vi "运维调试_五参数.vi"() -> ()   [LabVIEW 2016, in "斯坦道仪器.lvlib"]
uses:
  <vilib>/Utility/miscctls.llb/LVPointTypeDef.ctl
  PLC/PLC.lvlib
panel:
  in  "标样核查":bool
  in  "打开串口":bool
  in  "释放串口":bool
  in  "手动通电":bool
  out "多参数横条运行状态":T1(xcontrol)
  in  "数据区":i32(listbox)
  in  "探头选择":u16(ring)=9 items=["氨氮"=3, "水温"=9, "pH值"=10, "溶解氧"=11, "电导率"=12, "浊度"=13, "叶绿素a"=14, "藻密度"=15, "蓝绿藻"=16, "氧化还原电位"=17, "溶解氧%"=18, "盐度"=19]
  in  "测量数据区读取":bool
  in  "测量数据区":i32(listbox)
  in  "状态告警区读取":bool
  in  "状态告警区":i32(listbox)
  in  "自动校准":bool
  in  "读取KB":bool
  in  "写入KB":bool
  out "B":dbl caption="校准值B:"
  out "K":dbl caption="校准值K:"
  in  "校准区探头选择":u16(ring)=9 items=["氨氮"=3, "水温"=9, "pH值"=10, "溶解氧"=11, "电导率"=12, "浊度"=13, "叶绿素a"=14, "藻密度"=15, "蓝绿藻"=16, "氧化还原电位"=17, "溶解氧%"=18, "盐度"=19]
  in  "停止测量(单探)":bool
  in  "启动测量(单探)":bool
  in  "控制命令区探头选择":u16(ring)=9 items=["氨氮"=3, "水温"=9, "pH值"=10, "溶解氧"=11, "电导率"=12, "浊度"=13, "叶绿素a"=14, "藻密度"=15, "蓝绿藻"=16, "氧化还原电位"=17, "溶解氧%"=18, "盐度"=19]
  in  "同步时间":bool
  in  "初始化(清洗)":bool
  in  "停止测量(全部)":bool
  in  "启动测量(全部)":bool
  in  "关键参数区读取":bool
  in  "关键参数区":i32(listbox)
  in  "传感器参数读取":bool
  in  "传感器区":i32(listbox)
  in  "返回":bool
  in  "设置":bool
  out "运行状态":string
  out "开机状态":bool
  in  "停止":bool
  in  "水样测试":bool
  out "集成报警信息":string
  # "控制命令区"
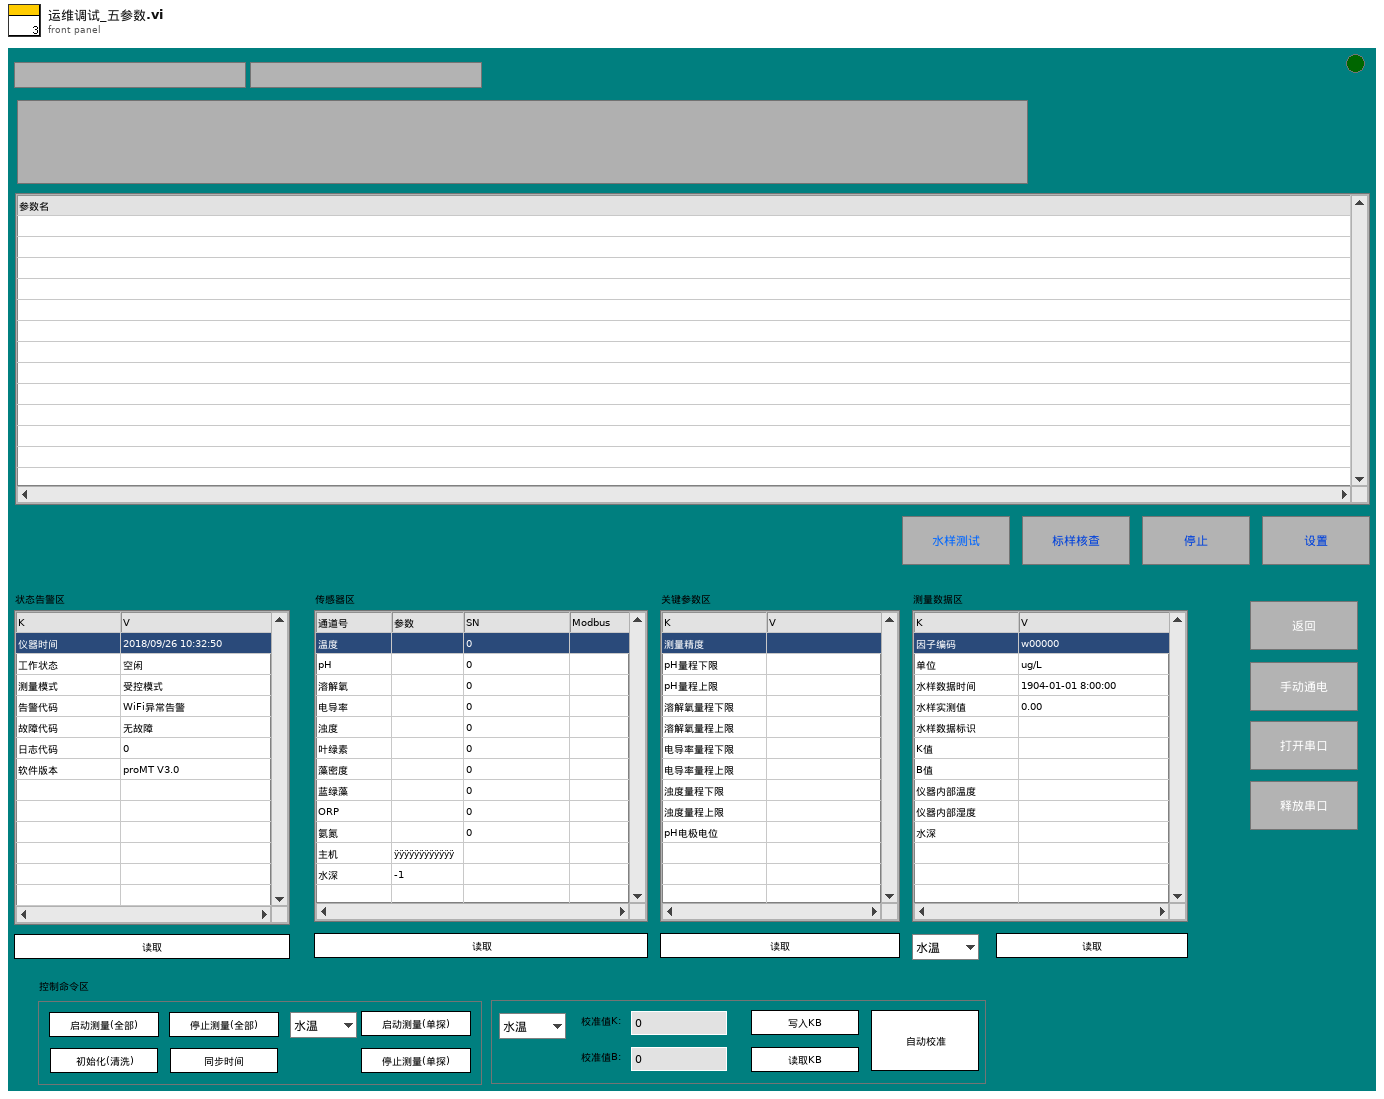
[diagram p1: front panel]
types:
  T1 = cluster{"系统时间":timestamp, "工作状态":u16, "测量模式":u16, "告警代码":enum16{"无告警", "缺试剂告警", "缺水样告警", "缺蒸馏水告警", "缺标液告警", "仪表漏液告警", "标定异常告警", "超量程告警", "加热异常", "低试剂预警", "超上限告警", "超下限告警", "仪表内部其他异常", "滴定异常告警", "电极异常告警", "量程切换告警", "参数设置告警", "PH电极电位异常", "电导率电极异常", "浊度光度异常", "溶解氧电极异常", "溶解氧光强异常", "温度异常告警", "PH异常告警", "溶解氧异常告警", "电导率异常告警", "浊度异常告警", "叶绿素异常告警", "藻密度异常告警", "蓝绿藻异常告警", "ORP异常告警", "氨氮异常告警", "清洁刷异常告警", "SD卡异常告警", "蓝牙异常告警", "Wifi异常告警", "流程异常告警"}, "故障代码":enum16{"无故障", "电机故障", "温度故障", "通讯故障", "滴定故障"}, "日志代码":u16, "软件版本":string}
  T2 = typedef "LVPointTypeDef.ctl" = cluster{"Horizontal":i16, "Vertical":i16}
  T3 = cluster{"时间标识":timestamp, "设备":string, "日志信息":string}
  T4 = enum16{"无告警", "缺试剂告警", "缺水样告警", "缺蒸馏水告警", "缺标液告警", "仪表漏液告警", "标定异常告警", "超量程告警", "加热异常", "低试剂预警", "超上限告警", "超下限告警", "仪表内部其他异常", "滴定异常告警", "电极异常告警", "量程切换告警", "参数设置告警", "PH电极电位异常", "电导率电极异常", "浊度光度异常", "溶解氧电极异常", "溶解氧光强异常", "温度异常告警", "PH异常告警", "溶解氧异常告警", "电导率异常告警", "浊度异常告警", "叶绿素异常告警", "藻密度异常告警", "蓝绿藻异常告警", "ORP异常告警", "氨氮异常告警", "清洁刷异常告警", "SD卡异常告警", "蓝牙异常告警", "Wifi异常告警", "流程异常告警"}
  T5 = cluster{"水温":dbl, "pH":dbl, "DO":dbl, "Cond":dbl, "Turb":dbl, "叶绿素":dbl, "藻密度":dbl, "蓝绿藻":dbl, "ORP":dbl, "NH3N":dbl}
  T6 = cluster{"因子编码":string, "单位":string, "标样参考值":sgl, "水样数据时间":timestamp, "水样实测值":sgl, "水样数据标识":string, "K":sgl, "B":sgl, "T":sgl, "H":sgl, "水深":sgl}
  T7 = enum8{"Enabled", "Disabled", "Disabled and Grayed Out"}
  T8 = cluster{"测量模式":enum16{"待机", "水样测试", "标样核查", "零点核查", "跨度核查", "空白测试", "平行样测试", "加标回收", "空白校准", "标样校准", "初始化（清洗）"}, "数据标记表":string, "测量时间":dbl}
  T9 = cluster{"测量模式":enum16{"待机", "水样测试", "标样核查", "零点核查", "跨度核查", "空白测试", "平行样测试", "加标回收", "空白校准", "标样校准", "初始化（清洗）"}, "数据标记表":string, "输出参数":cluster{"水温":bool, "pH":bool, "DO":bool, "浊度":bool, "电导率":bool, "保存组数":dbl}}
  T10 = enum16{"待机", "水样测试", "标样核查", "零点核查", "跨度核查", "空白测试", "平行样测试", "加标回收", "空白校准", "标样校准", "初始化（清洗）"}
  T11 = cluster{"starting address":u16, "holding register value":u16}
  T12 = enum16{"idle", "init", "读状态", "读参数", "多个写入", "单个写入", "线圈写入"}
  T13 = enum32{"Bad", "Idle", "Run top level", "Running"}
  T14 = cluster{"水温":bool, "pH":bool, "DO":bool, "浊度":bool, "电导率":bool, "保存组数":dbl}
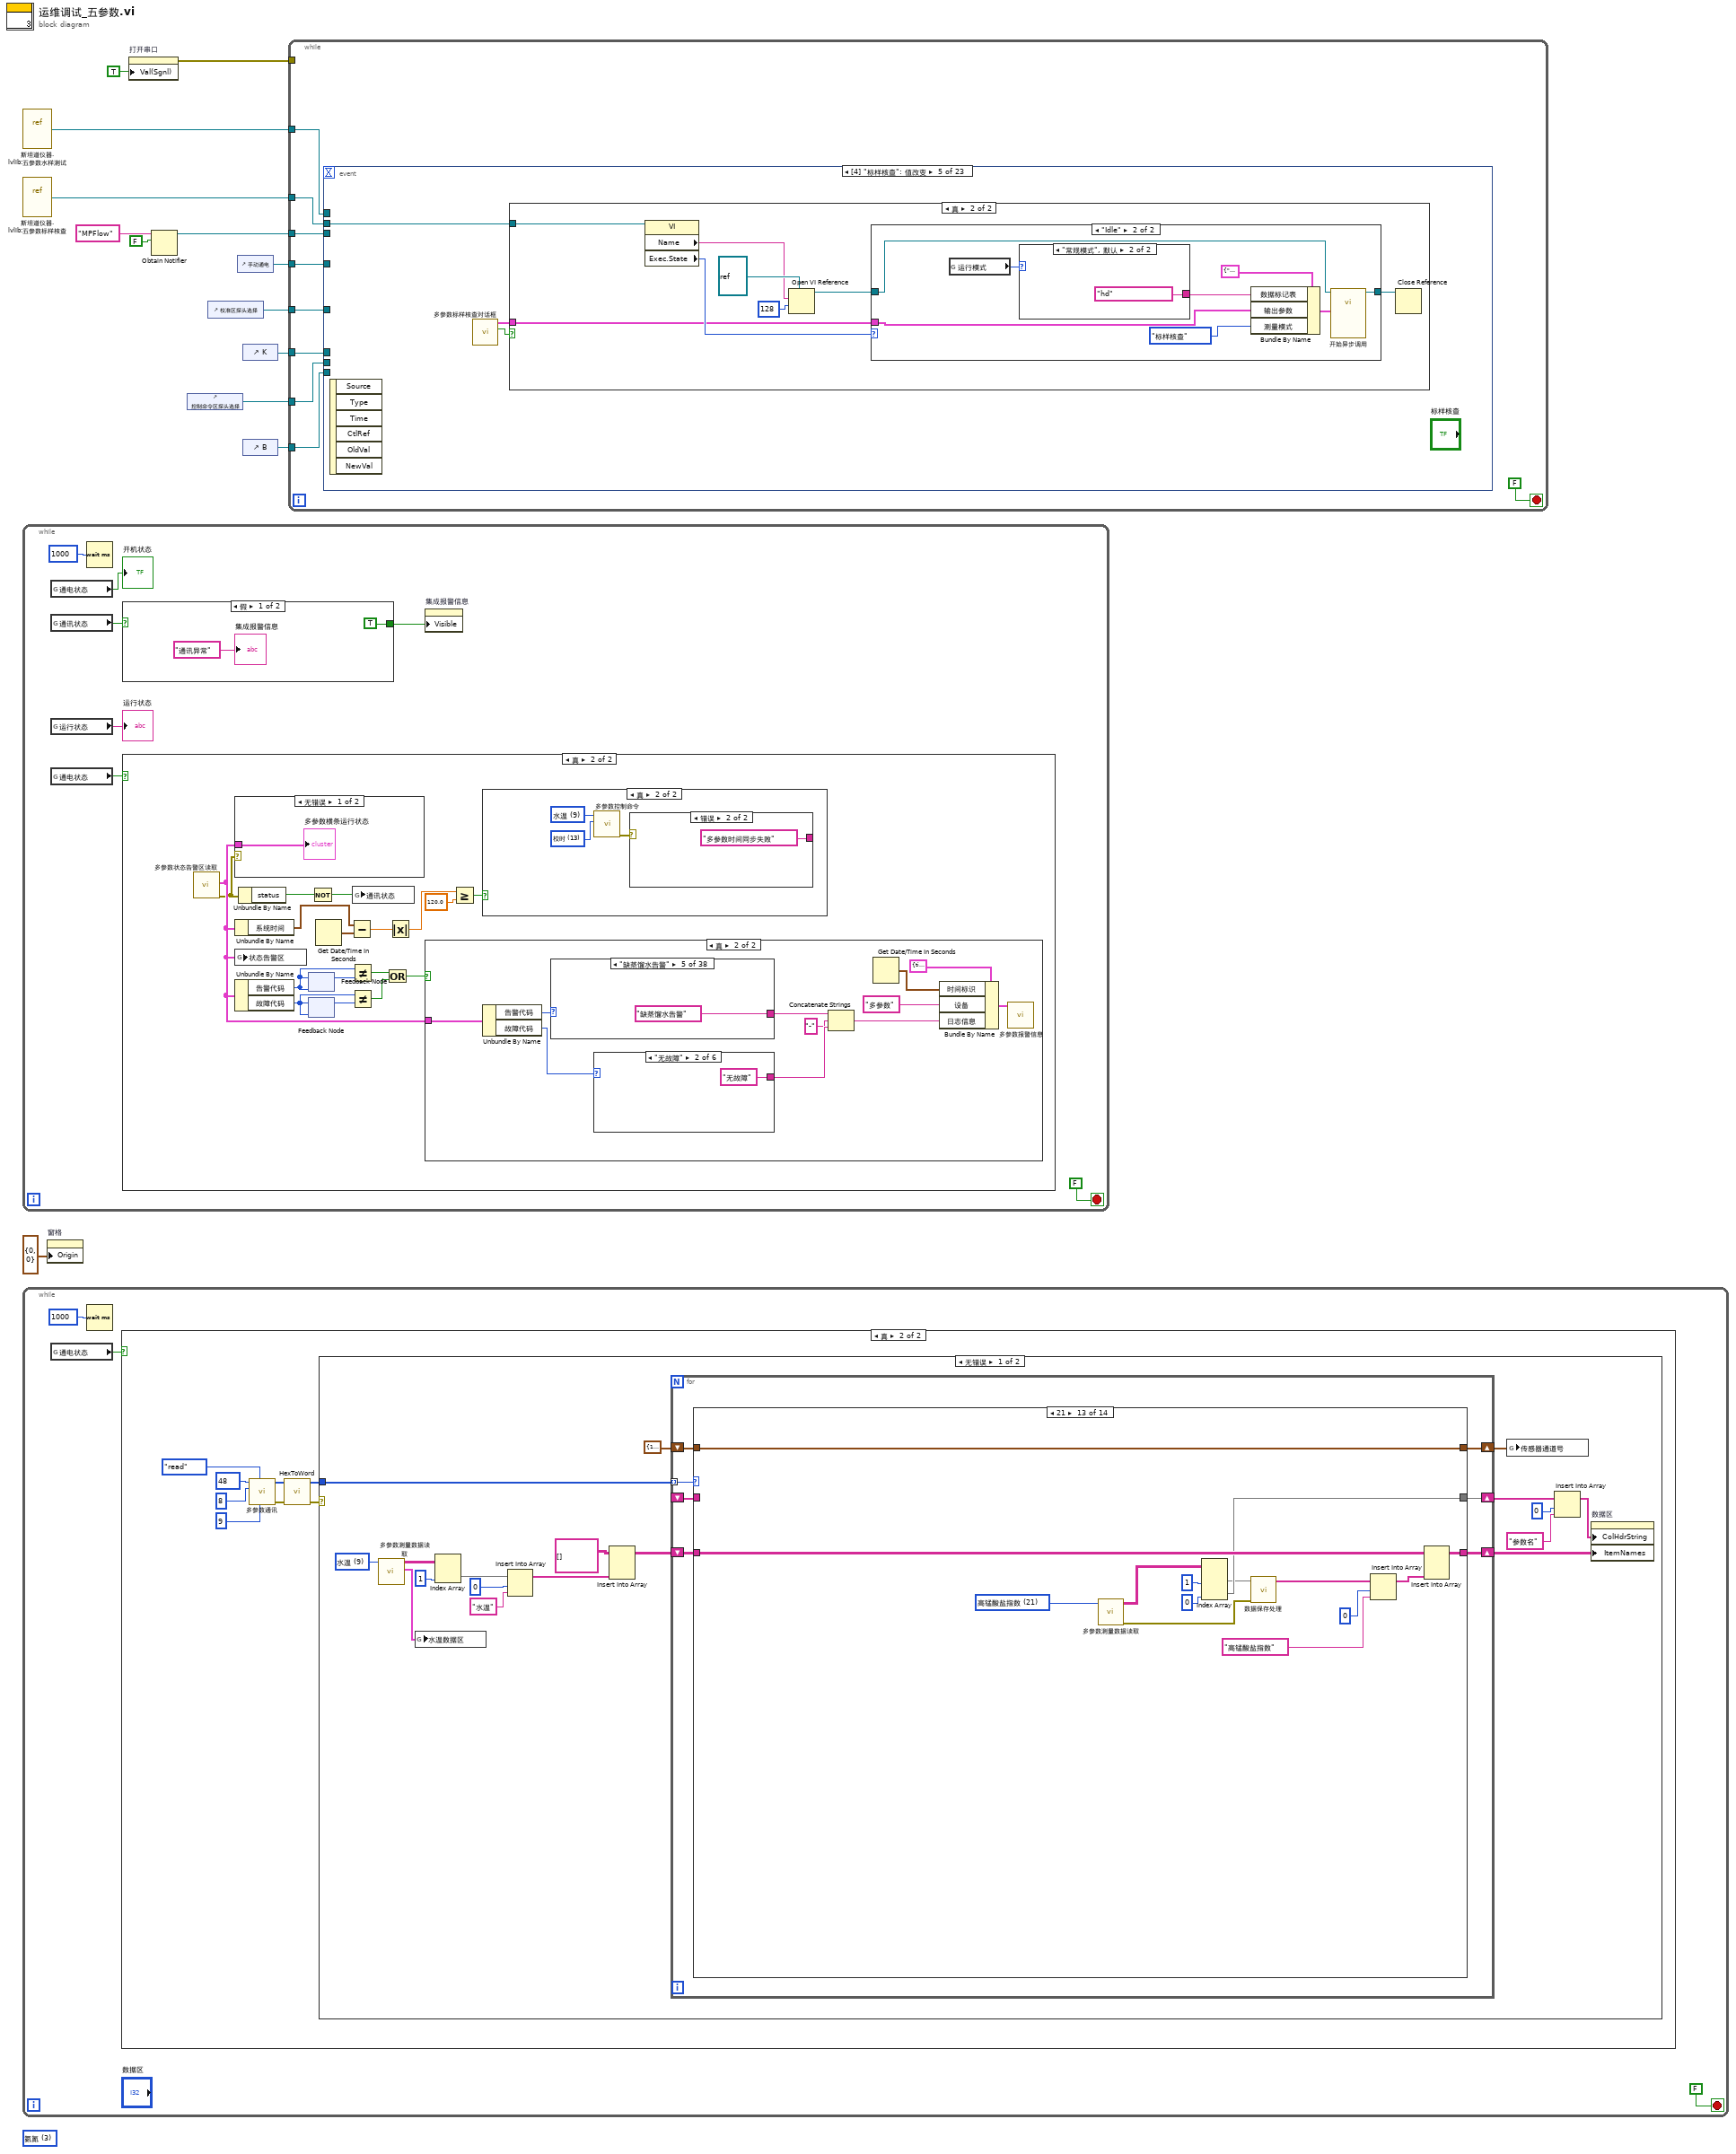
[diagram p0: block diagram]
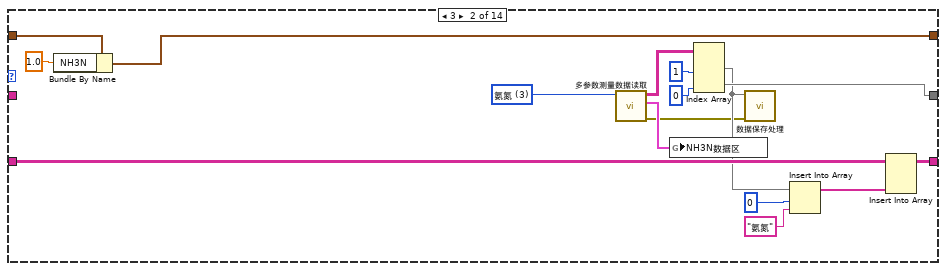
[diagram p4: hidden frame]
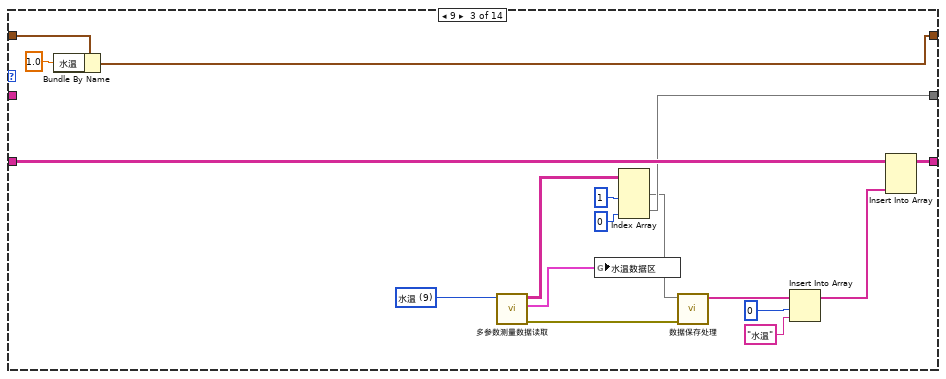
[diagram p5: hidden frame]
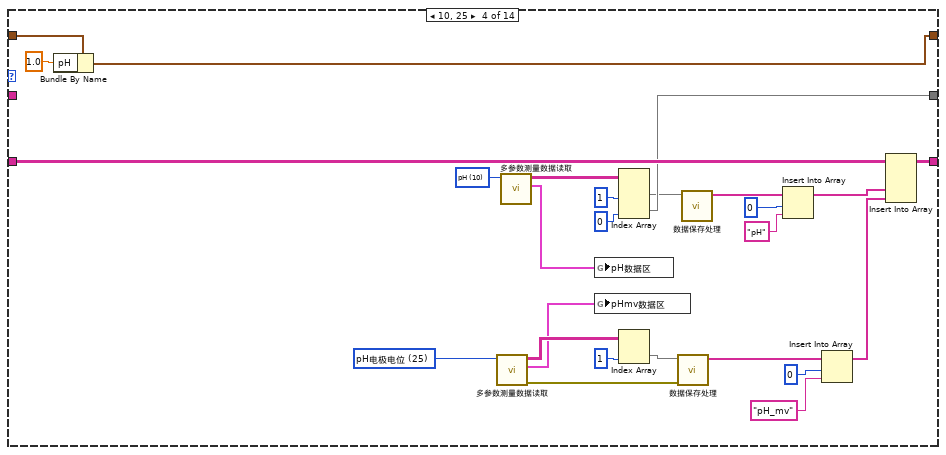
[diagram p6: hidden frame]
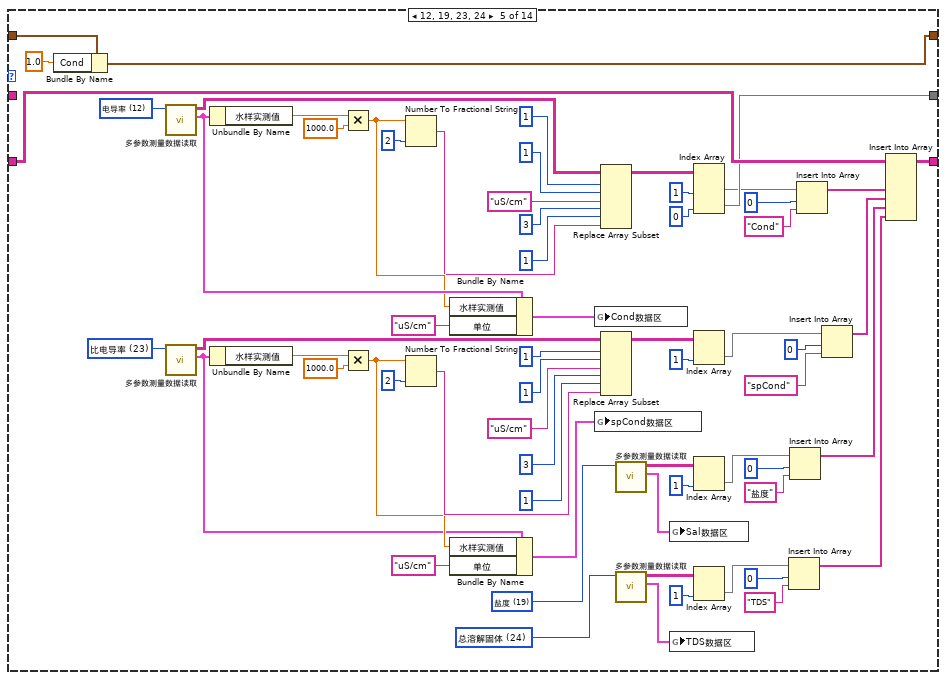
[diagram p7: hidden frame]
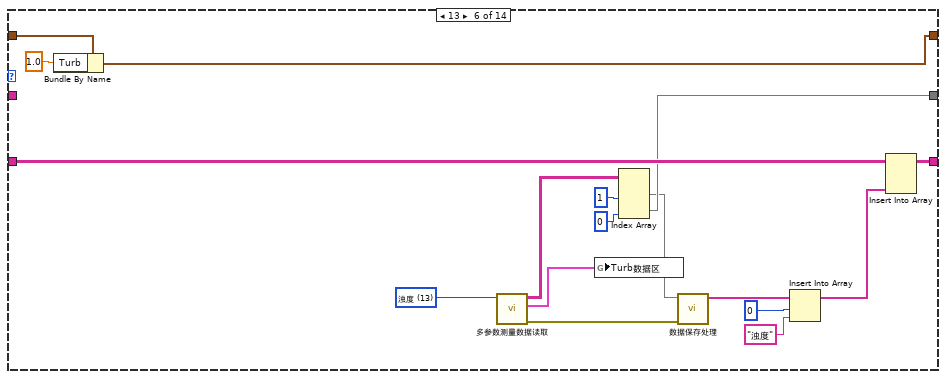
[diagram p8: hidden frame]
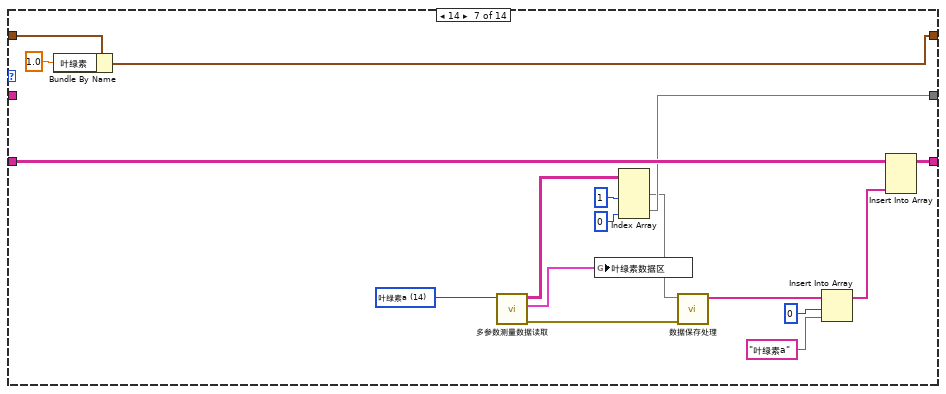
[diagram p9: hidden frame]
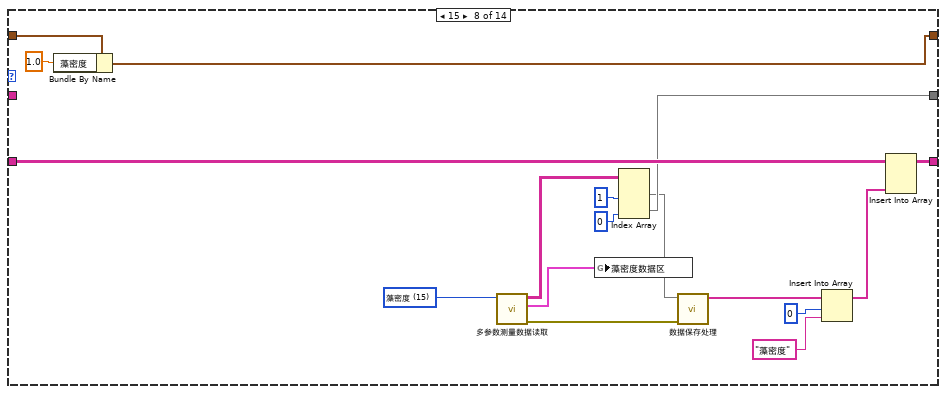
[diagram p10: hidden frame]
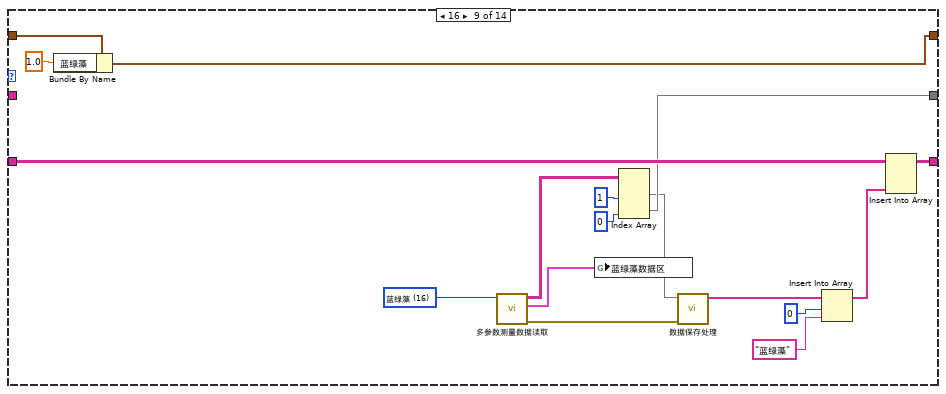
[diagram p11: hidden frame]
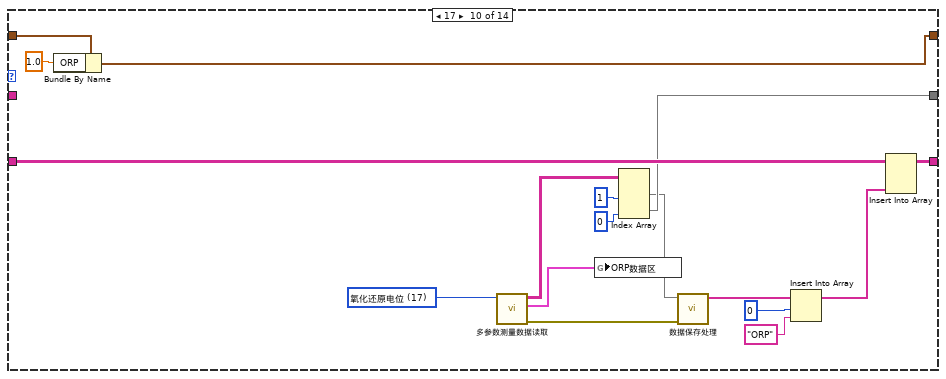
[diagram p12: hidden frame]
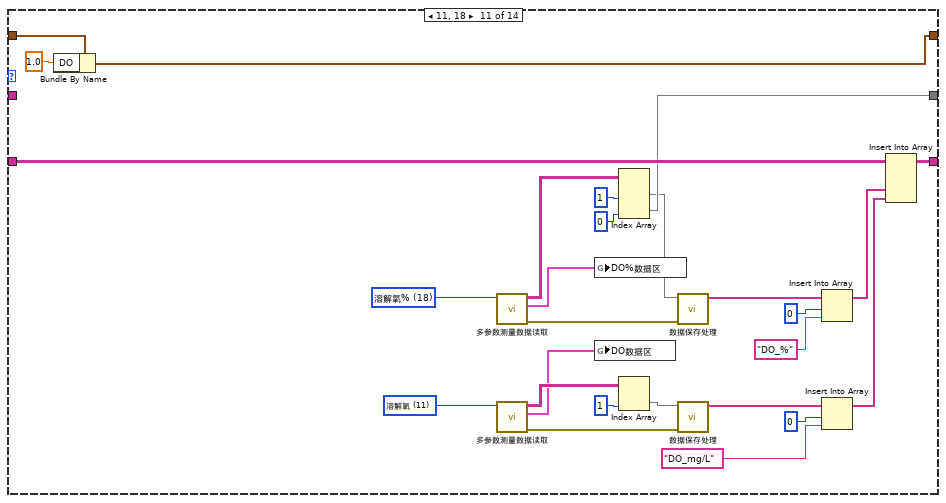
[diagram p13: hidden frame]
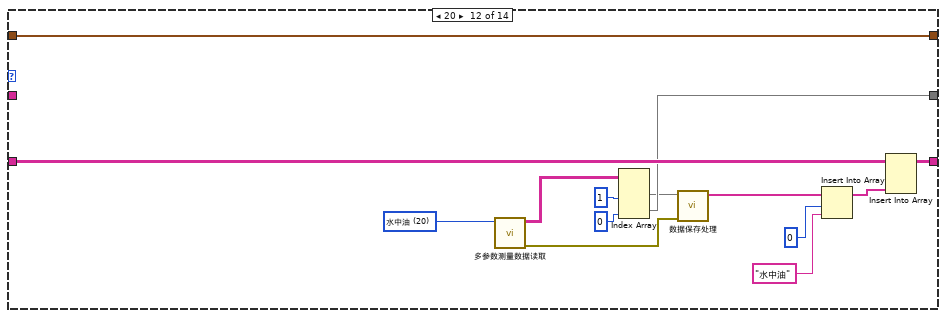
[diagram p14: hidden frame]
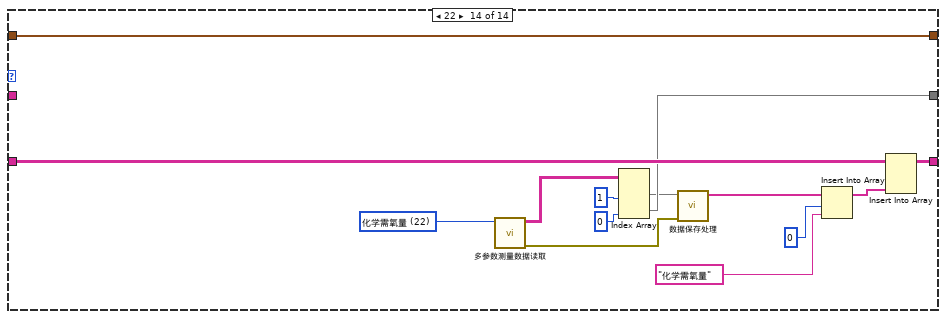
[diagram p15: hidden frame]
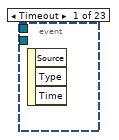
[diagram p17: hidden frame]
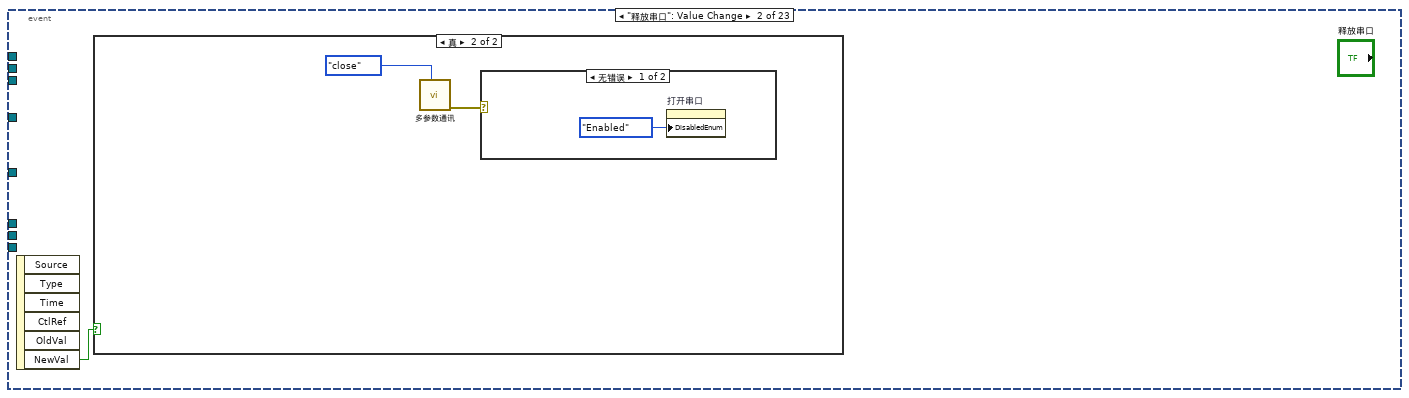
[diagram p18: hidden frame]
diagram:
  (unwired) u16 3 items=["氨氮"=3, "水温"=9, "pH"=10, "溶解氧"=11, "电导率"=12, "浊度"=13, "叶绿素a"=14, "藻密度"=15, "蓝绿藻"=16, "氧化还原电位"=17, "溶解氧%"=18, "盐度"=19, "水中油"=20, "高锰酸盐指数"=21, "化学需氧量"=22, "比电导率"=23, "总溶解固体"=24, "pH电极电位"=25] ("下拉列表")
  n1 = vi-ref "斯坦道仪器.lvlib:五参数水样测试.vi"() -> (w10:refnum<vi>)
  n2 = vi-ref "斯坦道仪器.lvlib:五参数标样核查.vi"() -> (w1:refnum<vi>)
  n3 = while {
    stop <- FALSE stop-if-true
    n4 = global read "多参数全局变量.vi" "通电状态"() -> (→"开机状态":bool)
    n5 = global read "多参数全局变量.vi" "通讯状态"() -> (w18:bool)
    n6 = global read "多参数全局变量.vi" "运行状态"() -> (→"运行状态":string)
    n7 = global read "多参数全局变量.vi" "通电状态"() -> (w14:bool)
    n8 = Wait (ms)(milliseconds to wait=u32 1000 ("等待时间（毫秒）")) -> ()  [unwired: 1 out]
    n9 = case shown="假" w18 {
      tunnel: [TRUE ("可见") _] -> w17
      frame False {
        "集成报警信息" <- "通讯异常" ("集成报警信息")
      }
      frame True {
      }
    }
    n10 = case shown="真" w14 {
      frame False {
      }
      frame True {
        n11 = call "多参数状态告警区读取.vi"() -> ("error out"=w21:errorcluster, "状态告警块"=w28:T1)  [unwired: 9 in, 1 out]
        n12 = case shown="无错误" w21 {
          tunnel: w28 -> [w38 _]
          frame No Error {
            "多参数横条运行状态" <- w38
          }
          frame Error {
          }
        }
        n13 = Unbundle By Name(w28) -> ("系统时间"=w27:timestamp)
        n14 = global write "多参数全局变量.vi" "状态告警区"(w28) -> ()
        n15 = Unbundle By Name(w28) -> ("告警代码"=w36:T4, "故障代码"=w34:enum16{"无故障", "电机故障", "温度故障", "通讯故障", "滴定故障"})
        n16 = Unbundle By Name(w21) -> ("status"=w30:bool)
        n17 = feedback #1(w36) -> (w37:T4)
        n18 = feedback-in #1(w36) -> ()
        n19 = feedback #2(w34) -> (w35:enum16{"无故障", "电机故障", "温度故障", "通讯故障", "滴定故障"})
        n20 = feedback-in #2(w34) -> ()
        n21 = Not(x=w30) -> (.not. x?=w29:bool)
        n22 = Get Date/Time In Seconds() -> (seconds since 1Jan1904=w26:timestamp)
        n23 = Subtract(x=w27, y=w26) -> (x-y=w25:dbl)
        n24 = Not Equal?(x=w36, y=w37) -> (x != y?=w32:bool)
        n25 = Not Equal?(x=w34, y=w35) -> (x != y?=w33:bool)
        n26 = global write "多参数全局变量.vi" "通讯状态"(w29) -> ()
        n27 = Or(x=w32, y=w33) -> (x .or. y?=w31:bool)
        n28 = Absolute Value(x=w25) -> (abs(x)=w24:dbl)
        n29 = case shown="真" w31 {
          tunnel: w28 -> [_ w54]
          frame False {
          }
          frame True {
            n30 = Unbundle By Name(w54) -> ("告警代码"=w53:T4, "故障代码"=w52:enum16{"无故障", "电机故障", "温度故障", "通讯故障", "滴定故障"})
            n31 = case shown="\"缺蒸馏水告警\"" w53 {
              selector: w53 -> [w65 _ _ _ _ _ _ _ _ _ _ _ _ _ _ _ _ _ _ _ _ _ _ _ _ _ _ _ _ _ _ _ _ _ _ _ _ _]
              tunnel: [w64 "无告警" "缺试剂告警" "缺水样告警" "缺蒸馏水告警" "缺标液告警" "仪表漏液告警" "标定异常告警" "超量程告警" "加热异常" "低试剂预警" "超上限告警" "超下限告警" "仪表内部其他异常" "滴定异常告警" "电极异常告警" "量程切换告警" "参数设置告警" "PH电极电位异常" "电导率电极异常" "浊度光度异常" "溶解氧电极异常" "溶解氧光强异常" "温度异常告警" "PH异常告警" "溶解氧异常告警" "电导率异常告警" "浊度异常告警" "叶绿素异常告警" "藻密度异常告警" "蓝绿藻异常告警" "ORP异常告警" "氨氮异常告警" "清洁刷异常告警" "SD卡异常告警" "蓝牙异常告警" "WiFi异常告警" "流程异常告警"] -> w51
              frame Default {
                n32 = Format Into String(format string="%d" ("格式字符串"), initial string="未知" ("工作状态"), w65) -> (resulting string=w64:string)  [unwired: 1 in, 1 out]
              }
              frame "无告警" {
              }
              frame "缺试剂告警" {
              }
              frame "缺水样告警" {
              }
              frame "缺蒸馏水告警" {
              }
              frame "缺标液告警" {
              }
              frame "仪表漏液告警" {
              }
              frame "标定异常告警" {
              }
              frame "超量程告警" {
              }
              frame "加热异常" {
              }
              frame "低试剂预警" {
              }
              frame "超上限告警" {
              }
              frame "超下限告警" {
              }
              frame "仪表内部其他异常" {
              }
              frame "滴定异常告警" {
              }
              frame "电极异常告警" {
              }
              frame "量程切换告警" {
              }
              frame "参数设置告警" {
              }
              frame "PH电极电位异常" {
              }
              frame "电导率电极异常" {
              }
              frame "浊度光度异常" {
              }
              frame "溶解氧电极异常" {
              }
              frame "溶解氧光强异常" {
              }
              frame "温度异常告警" {
              }
              frame "PH异常告警" {
              }
              frame "溶解氧异常告警" {
              }
              frame "电导率异常告警" {
              }
              frame "浊度异常告警" {
              }
              frame "叶绿素异常告警" {
              }
              frame "藻密度异常告警" {
              }
              frame "蓝绿藻异常告警" {
              }
              frame "ORP异常告警" {
              }
              frame "氨氮异常告警" {
              }
              frame "清洁刷异常告警" {
              }
              frame "SD卡异常告警" {
              }
              frame "蓝牙异常告警" {
              }
              frame "Wifi异常告警" {
              }
              frame "流程异常告警" {
              }
            }
            n33 = case shown="\"无故障\"" w52 {
              selector: w52 -> [w56 _ _ _ _ _]
              tunnel: [w55 "无故障" "电机故障" "温度故障" "通讯故障" "滴定故障"] -> w50
              frame Default {
                n34 = Format Into String(format string="%d" ("格式字符串"), initial string="未知" ("工作状态"), w56) -> (resulting string=w55:string)  [unwired: 1 in, 1 out]
              }
              frame "无故障" {
              }
              frame "电机故障" {
              }
              frame "温度故障" {
              }
              frame "通讯故障" {
              }
              frame "滴定故障" {
              }
            }
            n35 = Concatenate Strings(w51, "-" ("字符串"), w50) -> (w46:string)
            n36 = Get Date/Time In Seconds() -> (seconds since 1Jan1904=w45:timestamp)
            n37 = Bundle By Name(cluster=T3 {"时间标识"=timestamp(0 s since 1904-01-01), "设备"="", "日志信息"=""} ("data in"), "时间标识"=w45, "设备"="多参数", "日志信息"=w46) -> (w47:T3)
            n38 = call "多参数报警信息.vi"("data in"=w47) -> ()  [unwired: 10 in, 1 out]
          }
        }
        n39 = Greater Or Equal?(x=w24, y=120.0) -> (x >= y?=w23:bool)
        n40 = case shown="真" w23 {
          frame False {
          }
          frame True {
            w39 = u16 13 items=["启动测量（全部）"=1, "初始化（清洗）"=10, "停止测量（全部）"=11, "校时"=13, "启动测量（单个传感器）"=19, "停止测量（单个传感器）"=20] ("控制命令")
            w40 = u16 9 items=["氨氮"=3, "水温"=9, "pH值"=10, "溶解氧"=11, "电导率"=12, "浊度"=13, "叶绿素a"=14, "藻密度"=15, "蓝绿藻"=16, "氧化还原电位"=17, "溶解氧%"=18, "盐度"=19] ("站号")
            n41 = call "多参数控制命令.vi"("控制命令"=w39, "站号"=w40) -> ("error out"=w41:errorcluster)  [unwired: 9 in]
            n42 = case shown="错误" w41 {
              tunnel: ["多参数时间同步成功" ("消息") "多参数时间同步失败" ("消息")] -> _
              frame No Error {
              }
              frame Error {
              }
            }
          }
        }
      }
    }
    n43 = property on="集成报警信息" class="Str"("Visible"=w17) -> ()  [unwired: 2 in, 2 out]
  }
  n44 = while {
    stop <- FALSE stop-if-true
    n45 = global read "多参数全局变量.vi" "通电状态"() -> (w107:bool)
    n46 = Wait (ms)(milliseconds to wait=u32 1000 ("等待时间（毫秒）")) -> ()  [unwired: 1 out]
    n47 = case shown="真" w107 {
      frame False {
      }
      frame True {
        n48 = call "多参数通讯.vi"("Slave ID"=u8 9, "STEP"=enum16{"open", "read", "write", "close"}."read", "quantity"=u16 8, "starting address"=u16 48) -> ("error out"=w112:errorcluster, "Registers"=w113:u16[])  [unwired: 5 in, 1 out]
        n49 = call "HexToWord.vi"("数组"=w113) -> ("WORD"=w116:u16[])  [unwired: 10 in]
        n50 = case shown="无错误" w112 {
          tunnel: w116 -> [w131 _]
          frame No Error {
            w128 = u16 9 items=["氨氮"=3, "水温"=9, "pH"=10, "溶解氧"=11, "电导率"=12, "浊度"=13, "叶绿素a"=14, "藻密度"=15, "蓝绿藻"=16, "氧化还原电位"=17, "溶解氧%"=18, "盐度"=19, "水中油"=20, "高锰酸盐指数"=21, "化学需氧量"=22, "比电导率"=23, "总溶解固体"=24, "pH电极电位"=25] ("下拉列表")
            n51 = call "多参数测量数据读取.vi"("探头选择"=w128) -> ("测量数据块"=w117:T6, "添加的数组"=w127:string[][])  [unwired: 8 in, 1 out]
            n52 = global write "多参数全局变量.vi" "水温数据区"(w117) -> ()
            n53 = Index Array(array=w127, index (col)=1 ("禁用的索引 (列)")) -> (element=w122:string[])  [unwired: 1 in]
            n54 = Insert Into Array(array=w122, index=0 ("索引"), new element="水温") -> (w124:string[])
            n55 = Insert Into Array(array=string[][] [] ("子数组"), new element=w124) -> (w120:string[][])  [unwired: 2 in]
            n56 = for {
              tunnel: w131 -> [w141] mode=indexing
              shift-right: [w139] -> w129
              shift-left: w120 -> [w140]
              shift-right: [w138] -> w130
              shift-left: _ -> [w137]
              shift-right: [w136] -> w118
              shift-left: T5 {"水温"=1.0, "pH"=0.0, "DO"=0.0, "Cond"=0.0, "Turb"=0.0, "叶绿素"=0.0, "藻密度"=0.0, "蓝绿藻"=0.0, "ORP"=0.0, "NH3N"=0.0} ("传感器通道号") -> [w135]
              n57 = case shown="21" w141 {
                tunnel: w140 -> [w144 w156 w173 w199 w265 w281 w298 w315 w332 w349 w376 w390 w404 w418]
                tunnel: [w144 w155 w172 w198 w264 w280 w297 w314 w331 w348 w375 w389 w403 w417] -> w139
                tunnel: [w143 w153 w170 w196 w262 w278 w295 w312 w329 w346 w373 w387 w401 w415] -> w138
                tunnel: w137 -> [w143 _ _ _ _ _ _ _ _ _ _ _ _ _]
                tunnel: [w142 w148 w165 w185 w238 w273 w290 w307 w324 w341 w362 w384 w398 w412] -> w136
                tunnel: w135 -> [w142 w150 w167 w187 w239 w274 w291 w308 w325 w342 w363 w384 w398 w412]
                frame 0, Default {
                }
                frame 3 {
                  w160 = u16 3 items=["氨氮"=3, "水温"=9, "pH"=10, "溶解氧"=11, "电导率"=12, "浊度"=13, "叶绿素a"=14, "藻密度"=15, "蓝绿藻"=16, "氧化还原电位"=17, "溶解氧%"=18, "盐度"=19, "水中油"=20, "高锰酸盐指数"=21, "化学需氧量"=22, "比电导率"=23, "总溶解固体"=24, "pH电极电位"=25] ("下拉列表")
                  n58 = Bundle By Name(cluster=w150, "NH3N"=1.0) -> (w148:T5)
                  n59 = call "多参数测量数据读取.vi"("探头选择"=w160) -> ("error out"=w145:errorcluster, "测量数据块"=w147:T6, "添加的数组"=w159:string[][])  [unwired: 8 in]
                  n60 = global write "多参数全局变量.vi" "NH3N数据区"(w147) -> ()
                  n61 = Index Array(array=w159, index (col) #1=1 ("禁用的索引 (列)"), index (col) #2=0 ("禁用的索引 (列)")) -> (element #1=w146:string[], element #2=w153:string[])  [unwired: 2 in]
                  n62 = call "数据保存处理.vi"("error in (no error)"=w145, "数组"=w146) -> ()  [unwired: 8 in, 2 out]
                  n63 = Insert Into Array(array=w146, index=0 ("索引"), new element="氨氮") -> (w154:string[])
                  n64 = Insert Into Array(array=w156, new element=w154) -> (w155:string[][])  [unwired: 2 in]
                }
                frame 9 {
                  w177 = u16 9 items=["氨氮"=3, "水温"=9, "pH"=10, "溶解氧"=11, "电导率"=12, "浊度"=13, "叶绿素a"=14, "藻密度"=15, "蓝绿藻"=16, "氧化还原电位"=17, "溶解氧%"=18, "盐度"=19, "水中油"=20, "高锰酸盐指数"=21, "化学需氧量"=22, "比电导率"=23, "总溶解固体"=24, "pH电极电位"=25] ("下拉列表")
                  n65 = Bundle By Name(cluster=w167, "水温"=1.0) -> (w165:T5)
                  n66 = call "多参数测量数据读取.vi"("探头选择"=w177) -> ("error out"=w161:errorcluster, "测量数据块"=w164:T6, "添加的数组"=w176:string[][])  [unwired: 8 in]
                  n67 = global write "多参数全局变量.vi" "水温数据区"(w164) -> ()
                  n68 = Index Array(array=w176, index (col) #1=1 ("禁用的索引 (列)"), index (col) #2=0 ("禁用的索引 (列)")) -> (element #1=w163:string[], element #2=w170:string[])  [unwired: 2 in]
                  n69 = call "数据保存处理.vi"("error in (no error)"=w161, "数组"=w163) -> ("数组 2"=w162:string[])  [unwired: 8 in, 1 out]
                  n70 = Insert Into Array(array=w162, index=0 ("索引"), new element="水温") -> (w171:string[])
                  n71 = Insert Into Array(array=w173, new element=w171) -> (w172:string[][])  [unwired: 2 in]
                }
                frame 10, 25 {
                  w189 = u16 25 items=["氨氮"=3, "水温"=9, "pH"=10, "溶解氧"=11, "电导率"=12, "浊度"=13, "叶绿素a"=14, "藻密度"=15, "蓝绿藻"=16, "氧化还原电位"=17, "溶解氧%"=18, "盐度"=19, "水中油"=20, "高锰酸盐指数"=21, "化学需氧量"=22, "比电导率"=23, "总溶解固体"=24, "pH电极电位"=25] ("下拉列表")
                  w203 = u16 10 items=["氨氮"=3, "水温"=9, "pH"=10, "溶解氧"=11, "电导率"=12, "浊度"=13, "叶绿素a"=14, "藻密度"=15, "蓝绿藻"=16, "氧化还原电位"=17, "溶解氧%"=18, "盐度"=19, "水中油"=20, "高锰酸盐指数"=21, "化学需氧量"=22, "比电导率"=23, "总溶解固体"=24, "pH电极电位"=25] ("下拉列表")
                  n72 = Bundle By Name(cluster=w187, "pH"=1.0) -> (w185:T5)
                  n73 = call "多参数测量数据读取.vi"("探头选择"=w189) -> ("error out"=w182:errorcluster, "测量数据块"=w183:T6, "添加的数组"=w190:string[][])  [unwired: 8 in]
                  n74 = call "多参数测量数据读取.vi"("探头选择"=w203) -> ("测量数据块"=w184:T6, "添加的数组"=w202:string[][])  [unwired: 8 in, 1 out]
                  n75 = global write "多参数全局变量.vi" "pH数据区"(w184) -> ()
                  n76 = global write "多参数全局变量.vi" "pHmv数据区"(w183) -> ()
                  n77 = Index Array(array=w202, index (col) #1=1 ("禁用的索引 (列)"), index (col) #2=0 ("禁用的索引 (列)")) -> (element #1=w179:string[], element #2=w196:string[])  [unwired: 2 in]
                  n78 = Index Array(array=w190, index (col)=1 ("禁用的索引 (列)")) -> (element=w181:string[])  [unwired: 1 in]
                  n79 = call "数据保存处理.vi"("error in (no error)"=w182, "数组"=w181) -> ("数组 2"=w180:string[])  [unwired: 8 in, 1 out]
                  n80 = call "数据保存处理.vi"("数组"=w179) -> ("数组 2"=w178:string[])  [unwired: 9 in, 1 out]
                  n81 = Insert Into Array(array=w178, index=0 ("索引"), new element="pH") -> (w197:string[])
                  n82 = Insert Into Array(array=w180, index=0 ("索引"), new element="pH_mv") -> (w188:string[])
                  n83 = Insert Into Array(array=w199, new element #1=w197, new element #2=w188) -> (w198:string[][])  [unwired: 2 in]
                }
                frame 12, 19, 23, 24 {
                  w242 = u16 24 items=["氨氮"=3, "水温"=9, "pH"=10, "溶解氧"=11, "电导率"=12, "浊度"=13, "叶绿素a"=14, "藻密度"=15, "蓝绿藻"=16, "氧化还原电位"=17, "溶解氧%"=18, "盐度"=19, "水中油"=20, "高锰酸盐指数"=21, "化学需氧量"=22, "比电导率"=23, "总溶解固体"=24, "pH电极电位"=25] ("下拉列表")
                  w254 = u16 19 items=["氨氮"=3, "水温"=9, "pH"=10, "溶解氧"=11, "电导率"=12, "浊度"=13, "叶绿素a"=14, "藻密度"=15, "蓝绿藻"=16, "氧化还原电位"=17, "溶解氧%"=18, "盐度"=19, "水中油"=20, "高锰酸盐指数"=21, "化学需氧量"=22, "比电导率"=23, "总溶解固体"=24, "pH电极电位"=25] ("下拉列表")
                  w256 = u16 23 items=["氨氮"=3, "水温"=9, "pH"=10, "溶解氧"=11, "电导率"=12, "浊度"=13, "叶绿素a"=14, "藻密度"=15, "蓝绿藻"=16, "氧化还原电位"=17, "溶解氧%"=18, "盐度"=19, "水中油"=20, "高锰酸盐指数"=21, "化学需氧量"=22, "比电导率"=23, "总溶解固体"=24, "pH电极电位"=25] ("下拉列表")
                  w268 = u16 12 items=["氨氮"=3, "水温"=9, "pH"=10, "溶解氧"=11, "电导率"=12, "浊度"=13, "叶绿素a"=14, "藻密度"=15, "蓝绿藻"=16, "氧化还原电位"=17, "溶解氧%"=18, "盐度"=19, "水中油"=20, "高锰酸盐指数"=21, "化学需氧量"=22, "比电导率"=23, "总溶解固体"=24, "pH电极电位"=25] ("下拉列表")
                  n84 = Bundle By Name(cluster=w239, "Cond"=1.0 ("DO")) -> (w238:T5)
                  n85 = call "多参数测量数据读取.vi"("探头选择"=w268) -> ("测量数据块"=w228:T6, "添加的数组"=w235:string[][])  [unwired: 8 in, 1 out]
                  n86 = call "多参数测量数据读取.vi"("探头选择"=w256) -> ("测量数据块"=w206:T6, "添加的数组"=w207:string[][])  [unwired: 8 in, 1 out]
                  n87 = Unbundle By Name(w228) -> ("水样实测值"=w230:sgl)
                  n88 = Unbundle By Name(w206) -> ("水样实测值"=w213:sgl)
                  n89 = Multiply(x=w230, y=sgl 1000.0) -> (x*y=w223:sgl)
                  n90 = Multiply(x=w213, y=sgl 1000.0) -> (x*y=w218:sgl)
                  n91 = Number To Fractional String(number=w223, precision (6)=i16 2 ("精度(6)")) -> (F-format string=w221:string)  [unwired: 2 in]
                  n92 = Number To Fractional String(number=w218, precision (6)=i16 2 ("精度(6)")) -> (F-format string=w220:string)  [unwired: 2 in]
                  n93 = Bundle By Name(cluster=w228, "水样实测值"=w223, "单位"="uS/cm" ("新元素/子数组")) -> (w226:T6)
                  n94 = Bundle By Name(cluster=w206, "水样实测值"=w218, "单位"="uS/cm" ("新元素/子数组")) -> (w205:T6)
                  n95 = global write "多参数全局变量.vi" "Cond数据区"(w226) -> ()
                  n96 = global write "多参数全局变量.vi" "spCond数据区"(w205) -> ()
                  n97 = Replace Array Subset(array=w235, new element #1="uS/cm" ("新元素/子数组"), index (row) #1=1 ("索引 (行)"), index (col) #1=1 ("禁用的索引 (列)"), new element #2=w221, index (row) #2=3 ("索引 (行)"), index (col) #2=1 ("禁用的索引 (列)")) -> (w231:string[][])
                  n98 = Replace Array Subset(array=w207, new element #1="uS/cm" ("新元素/子数组"), index (row) #1=1 ("索引 (行)"), index (col) #1=1 ("禁用的索引 (列)"), new element #2=w220, index (row) #2=3 ("索引 (行)"), index (col) #2=1 ("禁用的索引 (列)")) -> (w212:string[][])
                  n99 = call "多参数测量数据读取.vi"("探头选择"=w254) -> ("测量数据块"=w237:T6, "添加的数组"=w253:string[][])  [unwired: 8 in, 1 out]
                  n100 = call "多参数测量数据读取.vi"("探头选择"=w242) -> ("测量数据块"=w236:T6, "添加的数组"=w243:string[][])  [unwired: 8 in, 1 out]
                  n101 = global write "多参数全局变量.vi" "Sal数据区"(w237) -> ()
                  n102 = global write "多参数全局变量.vi" "TDS数据区"(w236) -> ()
                  n103 = Index Array(array=w231, index (col) #1=1 ("禁用的索引 (列)"), index (col) #2=0 ("禁用的索引 (列)")) -> (element #1=w259:string[], element #2=w262:string[])  [unwired: 2 in]
                  n104 = Index Array(array=w212, index (col)=1 ("禁用的索引 (列)")) -> (element=w204:string[])  [unwired: 1 in]
                  n105 = Index Array(array=w253, index (col)=1 ("禁用的索引 (列)")) -> (element=w249:string[])  [unwired: 1 in]
                  n106 = Index Array(array=w243, index (col)=1 ("禁用的索引 (列)")) -> (element=w247:string[])  [unwired: 1 in]
                  n107 = Insert Into Array(array=w247, index=0 ("索引"), new element="TDS") -> (w241:string[])
                  n108 = Insert Into Array(array=w249, index=0 ("索引"), new element="盐度") -> (w248:string[])
                  n109 = Insert Into Array(array=w259, index=0 ("索引"), new element="Cond") -> (w263:string[])
                  n110 = Insert Into Array(array=w204, index=0 ("索引"), new element="spCond") -> (w255:string[])
                  n111 = Insert Into Array(array=w265, new element #1=w263, new element #2=w255, new element #3=w248, new element #4=w241) -> (w264:string[][])  [unwired: 2 in]
                }
                frame 13 {
                  w285 = u16 13 items=["氨氮"=3, "水温"=9, "pH"=10, "溶解氧"=11, "电导率"=12, "浊度"=13, "叶绿素a"=14, "藻密度"=15, "蓝绿藻"=16, "氧化还原电位"=17, "溶解氧%"=18, "盐度"=19, "水中油"=20, "高锰酸盐指数"=21, "化学需氧量"=22, "比电导率"=23, "总溶解固体"=24, "pH电极电位"=25] ("下拉列表")
                  n112 = Bundle By Name(cluster=w274, "Turb"=1.0 ("DO")) -> (w273:T5)
                  n113 = call "多参数测量数据读取.vi"("探头选择"=w285) -> ("error out"=w271:errorcluster, "测量数据块"=w272:T6, "添加的数组"=w284:string[][])  [unwired: 8 in]
                  n114 = global write "多参数全局变量.vi" "Turb数据区"(w272) -> ()
                  n115 = Index Array(array=w284, index (col) #1=1 ("禁用的索引 (列)"), index (col) #2=0 ("禁用的索引 (列)")) -> (element #1=w270:string[], element #2=w278:string[])  [unwired: 2 in]
                  n116 = call "数据保存处理.vi"("error in (no error)"=w271, "数组"=w270) -> ("数组 2"=w269:string[])  [unwired: 8 in, 1 out]
                  n117 = Insert Into Array(array=w269, index=0 ("索引"), new element="浊度") -> (w279:string[])
                  n118 = Insert Into Array(array=w281, new element=w279) -> (w280:string[][])  [unwired: 2 in]
                }
                frame 14 {
                  w302 = u16 14 items=["氨氮"=3, "水温"=9, "pH"=10, "溶解氧"=11, "电导率"=12, "浊度"=13, "叶绿素a"=14, "藻密度"=15, "蓝绿藻"=16, "氧化还原电位"=17, "溶解氧%"=18, "盐度"=19, "水中油"=20, "高锰酸盐指数"=21, "化学需氧量"=22, "比电导率"=23, "总溶解固体"=24, "pH电极电位"=25] ("下拉列表")
                  n119 = Bundle By Name(cluster=w291, "叶绿素"=1.0 ("DO")) -> (w290:T5)
                  n120 = call "多参数测量数据读取.vi"("探头选择"=w302) -> ("error out"=w288:errorcluster, "测量数据块"=w289:T6, "添加的数组"=w301:string[][])  [unwired: 8 in]
                  n121 = global write "多参数全局变量.vi" "叶绿素数据区"(w289) -> ()
                  n122 = Index Array(array=w301, index (col) #1=1 ("禁用的索引 (列)"), index (col) #2=0 ("禁用的索引 (列)")) -> (element #1=w287:string[], element #2=w295:string[])  [unwired: 2 in]
                  n123 = call "数据保存处理.vi"("error in (no error)"=w288, "数组"=w287) -> ("数组 2"=w286:string[])  [unwired: 8 in, 1 out]
                  n124 = Insert Into Array(array=w286, index=0 ("索引"), new element="叶绿素a") -> (w296:string[])
                  n125 = Insert Into Array(array=w298, new element=w296) -> (w297:string[][])  [unwired: 2 in]
                }
                frame 15 {
                  w319 = u16 15 items=["氨氮"=3, "水温"=9, "pH"=10, "溶解氧"=11, "电导率"=12, "浊度"=13, "叶绿素a"=14, "藻密度"=15, "蓝绿藻"=16, "氧化还原电位"=17, "溶解氧%"=18, "盐度"=19, "水中油"=20, "高锰酸盐指数"=21, "化学需氧量"=22, "比电导率"=23, "总溶解固体"=24, "pH电极电位"=25] ("下拉列表")
                  n126 = Bundle By Name(cluster=w308, "藻密度"=1.0 ("DO")) -> (w307:T5)
                  n127 = call "多参数测量数据读取.vi"("探头选择"=w319) -> ("error out"=w305:errorcluster, "测量数据块"=w306:T6, "添加的数组"=w318:string[][])  [unwired: 8 in]
                  n128 = global write "多参数全局变量.vi" "藻密度数据区"(w306) -> ()
                  n129 = Index Array(array=w318, index (col) #1=1 ("禁用的索引 (列)"), index (col) #2=0 ("禁用的索引 (列)")) -> (element #1=w304:string[], element #2=w312:string[])  [unwired: 2 in]
                  n130 = call "数据保存处理.vi"("error in (no error)"=w305, "数组"=w304) -> ("数组 2"=w303:string[])  [unwired: 8 in, 1 out]
                  n131 = Insert Into Array(array=w303, index=0 ("索引"), new element="藻密度") -> (w313:string[])
                  n132 = Insert Into Array(array=w315, new element=w313) -> (w314:string[][])  [unwired: 2 in]
                }
                frame 16 {
                  w336 = u16 16 items=["氨氮"=3, "水温"=9, "pH"=10, "溶解氧"=11, "电导率"=12, "浊度"=13, "叶绿素a"=14, "藻密度"=15, "蓝绿藻"=16, "氧化还原电位"=17, "溶解氧%"=18, "盐度"=19, "水中油"=20, "高锰酸盐指数"=21, "化学需氧量"=22, "比电导率"=23, "总溶解固体"=24, "pH电极电位"=25] ("下拉列表")
                  n133 = Bundle By Name(cluster=w325, "蓝绿藻"=1.0 ("DO")) -> (w324:T5)
                  n134 = call "多参数测量数据读取.vi"("探头选择"=w336) -> ("error out"=w322:errorcluster, "测量数据块"=w323:T6, "添加的数组"=w335:string[][])  [unwired: 8 in]
                  n135 = global write "多参数全局变量.vi" "蓝绿藻数据区"(w323) -> ()
                  n136 = Index Array(array=w335, index (col) #1=1 ("禁用的索引 (列)"), index (col) #2=0 ("禁用的索引 (列)")) -> (element #1=w321:string[], element #2=w329:string[])  [unwired: 2 in]
                  n137 = call "数据保存处理.vi"("error in (no error)"=w322, "数组"=w321) -> ("数组 2"=w320:string[])  [unwired: 8 in, 1 out]
                  n138 = Insert Into Array(array=w320, index=0 ("索引"), new element="蓝绿藻") -> (w330:string[])
                  n139 = Insert Into Array(array=w332, new element=w330) -> (w331:string[][])  [unwired: 2 in]
                }
                frame 17 {
                  w353 = u16 17 items=["氨氮"=3, "水温"=9, "pH"=10, "溶解氧"=11, "电导率"=12, "浊度"=13, "叶绿素a"=14, "藻密度"=15, "蓝绿藻"=16, "氧化还原电位"=17, "溶解氧%"=18, "盐度"=19, "水中油"=20, "高锰酸盐指数"=21, "化学需氧量"=22, "比电导率"=23, "总溶解固体"=24, "pH电极电位"=25] ("下拉列表")
                  n140 = Bundle By Name(cluster=w342, "ORP"=1.0 ("DO")) -> (w341:T5)
                  n141 = call "多参数测量数据读取.vi"("探头选择"=w353) -> ("error out"=w339:errorcluster, "测量数据块"=w340:T6, "添加的数组"=w352:string[][])  [unwired: 8 in]
                  n142 = global write "多参数全局变量.vi" "ORP数据区"(w340) -> ()
                  n143 = Index Array(array=w352, index (col) #1=1 ("禁用的索引 (列)"), index (col) #2=0 ("禁用的索引 (列)")) -> (element #1=w338:string[], element #2=w346:string[])  [unwired: 2 in]
                  n144 = call "数据保存处理.vi"("error in (no error)"=w339, "数组"=w338) -> ("数组 2"=w337:string[])  [unwired: 8 in, 1 out]
                  n145 = Insert Into Array(array=w337, index=0 ("索引"), new element="ORP") -> (w347:string[])
                  n146 = Insert Into Array(array=w349, new element=w347) -> (w348:string[][])  [unwired: 2 in]
                }
                frame 11, 18 {
                  w366 = u16 11 items=["氨氮"=3, "水温"=9, "pH"=10, "溶解氧"=11, "电导率"=12, "浊度"=13, "叶绿素a"=14, "藻密度"=15, "蓝绿藻"=16, "氧化还原电位"=17, "溶解氧%"=18, "盐度"=19, "水中油"=20, "高锰酸盐指数"=21, "化学需氧量"=22, "比电导率"=23, "总溶解固体"=24, "pH电极电位"=25] ("下拉列表")
                  w380 = u16 18 items=["氨氮"=3, "水温"=9, "pH"=10, "溶解氧"=11, "电导率"=12, "浊度"=13, "叶绿素a"=14, "藻密度"=15, "蓝绿藻"=16, "氧化还原电位"=17, "溶解氧%"=18, "盐度"=19, "水中油"=20, "高锰酸盐指数"=21, "化学需氧量"=22, "比电导率"=23, "总溶解固体"=24, "pH电极电位"=25] ("下拉列表")
                  n147 = Bundle By Name(cluster=w363, "DO"=1.0) -> (w362:T5)
                  n148 = call "多参数测量数据读取.vi"("探头选择"=w380) -> ("error out"=w359:errorcluster, "测量数据块"=w361:T6, "添加的数组"=w379:string[][])  [unwired: 8 in]
                  n149 = call "多参数测量数据读取.vi"("探头选择"=w366) -> ("error out"=w356:errorcluster, "测量数据块"=w360:T6, "添加的数组"=w367:string[][])  [unwired: 8 in]
                  n150 = global write "多参数全局变量.vi" "DO%数据区"(w361) -> ()
                  n151 = global write "多参数全局变量.vi" "DO数据区"(w360) -> ()
                  n152 = Index Array(array=w379, index (col) #1=1 ("禁用的索引 (列)"), index (col) #2=0 ("禁用的索引 (列)")) -> (element #1=w358:string[], element #2=w373:string[])  [unwired: 2 in]
                  n153 = Index Array(array=w367, index (col)=1 ("禁用的索引 (列)")) -> (element=w355:string[])  [unwired: 1 in]
                  n154 = call "数据保存处理.vi"("error in (no error)"=w359, "数组"=w358) -> ("数组 2"=w357:string[])  [unwired: 8 in, 1 out]
                  n155 = call "数据保存处理.vi"("error in (no error)"=w356, "数组"=w355) -> ("数组 2"=w354:string[])  [unwired: 8 in, 1 out]
                  n156 = Insert Into Array(array=w357, index=0 ("索引"), new element="DO_%") -> (w374:string[])
                  n157 = Insert Into Array(array=w354, index=0 ("索引"), new element="DO_mg/L") -> (w365:string[])
                  n158 = Insert Into Array(array=w376, new element #1=w374, new element #2=w365) -> (w375:string[][])  [unwired: 2 in]
                }
                frame 20 {
                  w394 = u16 20 items=["氨氮"=3, "水温"=9, "pH"=10, "溶解氧"=11, "电导率"=12, "浊度"=13, "叶绿素a"=14, "藻密度"=15, "蓝绿藻"=16, "氧化还原电位"=17, "溶解氧%"=18, "盐度"=19, "水中油"=20, "高锰酸盐指数"=21, "化学需氧量"=22, "比电导率"=23, "总溶解固体"=24, "pH电极电位"=25] ("下拉列表")
                  n159 = call "多参数测量数据读取.vi"("探头选择"=w394) -> ("error out"=w383:errorcluster, "添加的数组"=w393:string[][])  [unwired: 8 in, 1 out]
                  n160 = Index Array(array=w393, index (col) #1=1 ("禁用的索引 (列)"), index (col) #2=0 ("禁用的索引 (列)")) -> (element #1=w382:string[], element #2=w387:string[])  [unwired: 2 in]
                  n161 = call "数据保存处理.vi"("error in (no error)"=w383, "数组"=w382) -> ("数组 2"=w381:string[])  [unwired: 8 in, 1 out]
                  n162 = Insert Into Array(array=w381, index=0 ("索引"), new element="水中油") -> (w388:string[])
                  n163 = Insert Into Array(array=w390, new element=w388) -> (w389:string[][])  [unwired: 2 in]
                }
                frame 21 {
                  w408 = u16 21 items=["氨氮"=3, "水温"=9, "pH"=10, "溶解氧"=11, "电导率"=12, "浊度"=13, "叶绿素a"=14, "藻密度"=15, "蓝绿藻"=16, "氧化还原电位"=17, "溶解氧%"=18, "盐度"=19, "水中油"=20, "高锰酸盐指数"=21, "化学需氧量"=22, "比电导率"=23, "总溶解固体"=24, "pH电极电位"=25] ("下拉列表")
                  n164 = call "多参数测量数据读取.vi"("探头选择"=w408) -> ("error out"=w397:errorcluster, "添加的数组"=w407:string[][])  [unwired: 8 in, 1 out]
                  n165 = Index Array(array=w407, index (col) #1=1 ("禁用的索引 (列)"), index (col) #2=0 ("禁用的索引 (列)")) -> (element #1=w396:string[], element #2=w401:string[])  [unwired: 2 in]
                  n166 = call "数据保存处理.vi"("error in (no error)"=w397, "数组"=w396) -> ("数组 2"=w395:string[])  [unwired: 8 in, 1 out]
                  n167 = Insert Into Array(array=w395, index=0 ("索引"), new element="高锰酸盐指数") -> (w402:string[])
                  n168 = Insert Into Array(array=w404, new element=w402) -> (w403:string[][])  [unwired: 2 in]
                }
                frame 22 {
                  w422 = u16 22 items=["氨氮"=3, "水温"=9, "pH"=10, "溶解氧"=11, "电导率"=12, "浊度"=13, "叶绿素a"=14, "藻密度"=15, "蓝绿藻"=16, "氧化还原电位"=17, "溶解氧%"=18, "盐度"=19, "水中油"=20, "高锰酸盐指数"=21, "化学需氧量"=22, "比电导率"=23, "总溶解固体"=24, "pH电极电位"=25] ("下拉列表")
                  n169 = call "多参数测量数据读取.vi"("探头选择"=w422) -> ("error out"=w411:errorcluster, "添加的数组"=w421:string[][])  [unwired: 8 in, 1 out]
                  n170 = Index Array(array=w421, index (col) #1=1 ("禁用的索引 (列)"), index (col) #2=0 ("禁用的索引 (列)")) -> (element #1=w410:string[], element #2=w415:string[])  [unwired: 2 in]
                  n171 = call "数据保存处理.vi"("error in (no error)"=w411, "数组"=w410) -> ("数组 2"=w409:string[])  [unwired: 8 in, 1 out]
                  n172 = Insert Into Array(array=w409, index=0 ("索引"), new element="化学需氧量") -> (w416:string[])
                  n173 = Insert Into Array(array=w418, new element=w416) -> (w417:string[][])  [unwired: 2 in]
                }
              }
            }
            n174 = global write "多参数全局变量.vi" "传感器通道号"(w118) -> ()
            n175 = Insert Into Array(array=w130, index=0 ("索引"), new element="参数名" ("新元素/子数组")) -> (w134:string[])
            n176 = property on="数据区" class="MCListbox (严格)"("ColHdrString"=w134, "ItemNames"=w129) -> ()  [unwired: 2 in, 2 out]
          }
          frame Error {
          }
        }
      }
    }
  }
  n177 = property on="窗格" class="Pane"("Origin"=T2 {"Horizontal"=0, "Vertical"=0} ("原点")) -> ()  [unwired: 2 in, 2 out]
  n178 = property on="打开串口" class="Bool (严格)"("Val(Sgnl)"=TRUE ("值(信号)")) -> (error out=w2:errorcluster)  [unwired: 2 in, 1 out]
  n179 = Obtain Notifier(name (unnamed)="MPFlow" ("名称（未命名）"), notification data type=FALSE) -> (notifier out=w9:refnum<notifier>)  [unwired: 2 in, 2 out]
  n180 = control-ref of="控制命令区探头选择"() -> (w8:refnum<vi>)
  n181 = control-ref of="校准区探头选择"() -> (w5:refnum<vi>)
  n182 = control-ref of="手动通电"() -> (w4:refnum<vi>)
  n183 = control-ref of="K"() -> (w7:refnum<vi>)
  n184 = control-ref of="B"() -> (w6:refnum<vi>)
  n185 = while {
    tunnel: w10 -> [w430]
    tunnel: w9 -> [w429]
    tunnel: w8 -> [w428]
    tunnel: w7 -> [w427]
    tunnel: w6 -> [w426]
    tunnel: w5 -> [w425]
    tunnel: w4 -> [w424]
    tunnel: w2 -> [_]
    tunnel: w1 -> [w423]
    stop <- FALSE stop-if-true
    n186 = event shown="[4] \"标样核查\": 值改变" {
      selector: _ -> [_ _ _ _ _ _ _ _ _ _ _ _ _ _ _ _ _ _ _ _ _ _ _]
      dyn-events: _ -> [_ _ _ _ _ _ _ _ _ _ _ _ _ _ _ _ _ _ _ _ _ _ _]
      timeout: _ -> [_ _ _ _ _ _ _ _ _ _ _ _ _ _ _ _ _ _ _ _ _ _ _]
      tunnel: w430 -> [_ _ _ w446 _ _ _ _ _ _ _ _ _ _ _ _ _ _ _ _ _ _ _]
      tunnel: w429 -> [_ _ _ _ _ w491 _ _ _ _ _ _ _ _ _ _ _ _ _ _ _ _ _]
      tunnel: w428 -> [_ _ _ _ _ _ _ _ _ _ _ _ _ _ _ _ w558 w569 _ _ _ _ _]
      tunnel: w427 -> [_ _ _ _ _ _ _ _ _ _ _ _ _ _ _ _ _ _ w580 _ _ _ _]
      tunnel: w426 -> [_ _ _ _ _ _ _ _ _ _ _ _ _ _ _ _ _ _ w582 _ _ _ _]
      tunnel: w425 -> [_ _ _ _ _ _ _ _ _ _ _ _ _ _ _ _ _ _ w584 _ w600 _ _]
      tunnel: w424 -> [_ _ _ _ _ _ _ _ w499 w504 w509 w515 w520 w529 w538 w547 w556 w567 w578 _ w598 w610 _]
      tunnel: w423 -> [_ _ _ _ w468 _ _ _ _ _ _ _ _ _ _ _ _ _ _ _ _ _ _]
      event Timeout {
        n187 = event-data() -> ()  [unwired: 1 in, 3 out]
      }
      event "释放串口": Value Change {
        n188 = event-data() -> ("NewVal"=w432:bool)  [unwired: 1 in, 5 out]
        n189 = case shown="真" w432 {
          frame False {
          }
          frame True {
            n190 = call "多参数通讯.vi"("STEP"=enum16{"open", "read", "write", "close"}."close") -> ("error out"=w433:errorcluster)  [unwired: 8 in, 2 out]
            n191 = case shown="无错误" w433 {
              frame No Error {
                n192 = property on="打开串口" class="Bool (严格)"("DisabledEnum"=T7."Enabled" ("禁用")) -> ()  [unwired: 2 in, 2 out]
              }
              frame Error {
              }
            }
          }
        }
      }
      event "打开串口": Value Change {
        n193 = event-data() -> ("NewVal"=w436:bool)  [unwired: 1 in, 5 out]
        n194 = case shown="真" w436 {
          frame False {
          }
          frame True {
            n195 = call "多参数通讯.vi"("STEP"=enum16{"open", "read", "write", "close"}."open") -> ("error out"=w437:errorcluster)  [unwired: 8 in, 2 out]
            n196 = case shown="错误" w437 {
              tunnel: [T7."Disabled and Grayed Out" ("禁用") T7."Enabled" ("禁用")] -> w439
              frame No Error {
              }
              frame Error {
                n197 = One Button Dialog(message="多参数串口打开失败" ("消息")) -> ()  [unwired: 1 in, 1 out]
              }
            }
            n198 = property on="打开串口" class="Bool (严格)"("DisabledEnum"=w439, "Value"=FALSE ("打开串口")) -> ()  [unwired: 2 in, 2 out]
          }
        }
      }
      event "水样测试": Value Change {
        n199 = event-data() -> ()  [unwired: 1 in, 6 out]
        n200 = call "多参数启动参数对话框.vi"() -> ("确认"=w445:bool, "测量时间"=w444:dbl)  [unwired: 10 in]
        n201 = case shown="真" w445 {
          tunnel: w446 -> [_ w448]
          tunnel: w444 -> [_ w447]
          frame False {
          }
          frame True {
            n202 = property class="VI"(reference=w448) -> ("Name"=w452:string, "Exec.State"=w450:T13)  [unwired: 1 in, 2 out]
            n203 = Open VI Reference(type specifier VI Refnum (for type only)=refnum<vi> refnum ("类型说明符VI引用句柄（仅用于类型）"), vi path=w452, options=128 ("选项")) -> (vi reference=w451:refnum<vi>)  [unwired: 3 in, 1 out]
            n204 = case shown="\"Idle\"" w450 {
              tunnel: w451 -> [w456 w463]
              tunnel: [w456 w462] -> w449
              tunnel: w447 -> [_ w457]
              frame "Bad", Default {
                n205 = One Button Dialog(message="仪器已经启动，无需重复启动" ("消息")) -> ()  [unwired: 1 in, 1 out]
              }
              frame "Idle" {
                n206 = global read "系统变量.vi" "运行模式"() -> (w459:enum16{"维护模式", "常规模式", "应急模式", "质控模式"})
                n207 = case shown="\"常规模式\", 默认" w459 {
                  tunnel: ["M" ("数据标记表") "hd" ("数据标记表")] -> w458
                  frame "维护模式" {
                  }
                  frame "常规模式", Default {
                  }
                }
                n208 = Bundle By Name(cluster=T8 {"测量模式"=enum."水样测试", "数据标记表"="", "测量时间"=0.0} ("启动参数"), "数据标记表"=w458, "测量时间"=w457) -> (w460:T8)
                n209 = call-by-ref "开始异步调用"(reference=w463, "启动参数"=w460) -> (reference out=w462:refnum<vi>)  [unwired: 12 in, 1 out]
              }
            }
            n210 = Close Reference(reference=w449) -> ()  [unwired: 1 in, 1 out]
          }
        }
      }
      event "标样核查": Value Change {
        n211 = event-data() -> ()  [unwired: 1 in, 6 out]
        n212 = call "多参数标样核查对话框.vi"() -> ("确认"=w467:bool, "输出参数"=w466:T14)  [unwired: 10 in]
        n213 = case shown="真" w467 {
          tunnel: w468 -> [_ w470]
          tunnel: w466 -> [_ w469]
          frame False {
          }
          frame True {
            n214 = property class="VI"(reference=w470) -> ("Name"=w474:string, "Exec.State"=w472:T13)  [unwired: 1 in, 2 out]
            n215 = Open VI Reference(type specifier VI Refnum (for type only)=refnum<vi> refnum ("类型说明符VI引用句柄（仅用于类型）"), vi path=w474, options=128 ("选项")) -> (vi reference=w473:refnum<vi>)  [unwired: 3 in, 1 out]
            n216 = case shown="\"Idle\"" w472 {
              tunnel: w473 -> [w478 w486]
              tunnel: [w478 w485] -> w471
              tunnel: w469 -> [_ w482]
              frame "Bad", Default {
                n217 = One Button Dialog(message="仪器已经启动，无需重复启动" ("消息")) -> ()  [unwired: 1 in, 1 out]
              }
              frame "Idle" {
                n218 = global read "系统变量.vi" "运行模式"() -> (w484:enum16{"维护模式", "常规模式", "应急模式", "质控模式"})
                n219 = case shown="\"常规模式\", 默认" w484 {
                  tunnel: ["M" ("数据标记表") "hd" ("数据标记表")] -> w483
                  frame "维护模式" {
                  }
                  frame "常规模式", Default {
                  }
                }
                n220 = Bundle By Name(cluster=T9 {"测量模式"=enum."待机", "数据标记表"="", "输出参数"={"水温"=FALSE, "pH"=FALSE, "DO"=FALSE, "浊度"=FALSE, "电导率"=FALSE, "保存组数"=0.0}} ("启动参数"), "数据标记表"=w483, "输出参数"=w482, "测量模式"=T10."标样核查") -> (w479:T9)
                n221 = call-by-ref "开始异步调用"(reference=w486, "启动参数"=w479) -> (reference out=w485:refnum<vi>)  [unwired: 12 in, 1 out]
              }
            }
            n222 = Close Reference(reference=w471) -> ()  [unwired: 1 in, 1 out]
          }
        }
      }
      event "停止": Value Change {
        n223 = event-data() -> ()  [unwired: 1 in, 6 out]
        n224 = Two Button Dialog(message="请再一次确认是否停止测量" ("消息")) -> (T button?=w489:bool)  [unwired: 2 in]
        n225 = case shown="真" w489 {
          tunnel: w491 -> [_ w494]
          frame False {
          }
          frame True {
            w492 = u16 11 items=["启动测量（全部）"=1, "初始化（清洗）"=10, "停止测量（全部）"=11, "校时"=13, "启动测量（单个传感器）"=19, "停止测量（单个传感器）"=20] ("控制命令")
            w493 = u16 10 items=["氨氮"=3, "水温"=9, "pH值"=10, "溶解氧"=11, "电导率"=12, "浊度"=13, "叶绿素a"=14, "藻密度"=15, "蓝绿藻"=16, "氧化还原电位"=17, "溶解氧%"=18, "盐度"=19] ("站号")
            n226 = Send Notification(notification=TRUE ("通知"), notifier=w494) -> ()  [unwired: 1 in, 2 out]
            n227 = call "多参数控制命令.vi"("控制命令"=w492, "站号"=w493) -> ()  [unwired: 9 in, 1 out]
          }
        }
      }
      event "设置": Value Change {
        n228 = event-data() -> ()  [unwired: 1 in, 6 out]
        n229 = property on="窗格" class="Pane"("Origin"=T2 {"Horizontal"=0, "Vertical"=528} ("原点")) -> ()  [unwired: 2 in, 2 out]
      }
      event "返回": Value Change {
        n230 = event-data() -> ()  [unwired: 1 in, 6 out]
        n231 = property on="窗格" class="Pane"("Origin"=T2 {"Horizontal"=0, "Vertical"=0} ("原点")) -> ()  [unwired: 2 in, 2 out]
      }
      event "传感器参数读取": Value Change {
        n232 = event-data() -> ()  [unwired: 1 in, 6 out]
        n233 = property class="Bool (严格)"(reference=w499) -> ("Value"=w498:bool)  [unwired: 1 in, 2 out]
        n234 = case shown="真" w498 {
          frame False {
            n235 = One Button Dialog(message="启动失败，请先通电" ("消息")) -> ()  [unwired: 1 in, 1 out]
          }
          frame True {
            n236 = call "多参数传感器参数读取.vi"() -> ("error out"=w501:errorcluster, "添加的数组"=w502:string[][])  [unwired: 10 in]
            n237 = call <vilib>:"General Error Handler.vi"("error in (no error)"=w501) -> ()  [unwired: 10 in, 5 out]
            n238 = property on="传感器区" class="MCListbox (严格)"("ItemNames"=w502) -> ()  [unwired: 2 in, 2 out]
          }
        }
      }
      event "关键参数区读取": Value Change {
        n239 = event-data() -> ()  [unwired: 1 in, 6 out]
        n240 = property class="Bool (严格)"(reference=w504) -> ("Value"=w503:bool)  [unwired: 1 in, 2 out]
        n241 = case shown="假" w503 {
          frame False {
            n242 = One Button Dialog(message="启动失败，请先通电" ("消息")) -> ()  [unwired: 1 in, 1 out]
          }
          frame True {
            n243 = call "多参数关键参数读取.vi"() -> ("error out"=w506:errorcluster, "添加的数组"=w507:string[][])  [unwired: 10 in]
            n244 = call <vilib>:"General Error Handler.vi"("error in (no error)"=w506) -> ()  [unwired: 10 in, 5 out]
            n245 = property on="关键参数区" class="MCListbox (严格)"("ItemNames"=w507) -> ()  [unwired: 2 in, 2 out]
          }
        }
      }
      event "测量数据区读取": Value Change {
        n246 = event-data() -> ()  [unwired: 1 in, 6 out]
        n247 = property class="Bool (严格)"(reference=w509) -> ("Value"=w508:bool)  [unwired: 1 in, 2 out]
        n248 = case shown="假" w508 {
          frame False {
            n249 = One Button Dialog(message="启动失败，请先通电" ("消息")) -> ()  [unwired: 1 in, 1 out]
          }
          frame True {
            n250 = call "多参数测量数据读取.vi"("探头选择"="探头选择") -> ("error out"=w512:errorcluster, "添加的数组"=w513:string[][])  [unwired: 8 in, 1 out]
            n251 = call <vilib>:"General Error Handler.vi"("error in (no error)"=w512) -> ()  [unwired: 10 in, 5 out]
            n252 = property on="测量数据区" class="MCListbox (严格)"("ItemNames"=w513) -> ()  [unwired: 2 in, 2 out]
          }
        }
      }
      event "状态告警区读取": Value Change {
        n253 = event-data() -> ()  [unwired: 1 in, 6 out]
        n254 = property class="Bool (严格)"(reference=w515) -> ("Value"=w514:bool)  [unwired: 1 in, 2 out]
        n255 = case shown="真" w514 {
          frame False {
            n256 = One Button Dialog(message="启动失败，请先通电" ("消息")) -> ()  [unwired: 1 in, 1 out]
          }
          frame True {
            n257 = call "多参数状态告警区读取.vi"() -> ("error out"=w517:errorcluster, "添加的数组"=w518:string[][])  [unwired: 9 in, 1 out]
            n258 = call <vilib>:"General Error Handler.vi"("error in (no error)"=w517) -> ()  [unwired: 10 in, 5 out]
            n259 = property on="状态告警区" class="MCListbox (严格)"("ItemNames"=w518) -> ()  [unwired: 2 in, 2 out]
          }
        }
      }
      event "同步时间": Value Change {
        n260 = event-data() -> ()  [unwired: 1 in, 6 out]
        n261 = property class="Bool (严格)"(reference=w520) -> ("Value"=w519:bool)  [unwired: 1 in, 2 out]
        n262 = case shown="假" w519 {
          frame False {
            n263 = One Button Dialog(message="启动失败，请先通电" ("消息")) -> ()  [unwired: 1 in, 1 out]
          }
          frame True {
            w522 = u16 13 items=["启动测量（全部）"=1, "初始化（清洗）"=10, "停止测量（全部）"=11, "校时"=13, "启动测量（单个传感器）"=19, "停止测量（单个传感器）"=20] ("控制命令")
            w523 = u16 9 items=["氨氮"=3, "水温"=9, "pH值"=10, "溶解氧"=11, "电导率"=12, "浊度"=13, "叶绿素a"=14, "藻密度"=15, "蓝绿藻"=16, "氧化还原电位"=17, "溶解氧%"=18, "盐度"=19] ("站号")
            n264 = call "多参数控制命令.vi"("控制命令"=w522, "站号"=w523) -> ("error out"=w525:errorcluster)  [unwired: 9 in]
            n265 = case shown="错误" w525 {
              tunnel: ["时间同步成功" ("消息") "时间同步失败" ("消息")] -> w524
              frame No Error {
              }
              frame Error {
              }
            }
            n266 = One Button Dialog(message=w524) -> ()  [unwired: 1 in, 1 out]
          }
        }
      }
      event "启动测量(全部)": Value Change {
        n267 = event-data() -> ()  [unwired: 1 in, 6 out]
        n268 = property class="Bool (严格)"(reference=w529) -> ("Value"=w528:bool)  [unwired: 1 in, 2 out]
        n269 = case shown="假" w528 {
          frame False {
            n270 = One Button Dialog(message="启动失败，请先通电" ("消息")) -> ()  [unwired: 1 in, 1 out]
          }
          frame True {
            w531 = u16 1 items=["启动测量（全部）"=1, "初始化（清洗）"=10, "停止测量（全部）"=11, "校时"=13, "启动测量（单个传感器）"=19, "停止测量（单个传感器）"=20] ("控制命令")
            w532 = u16 9 items=["氨氮"=3, "水温"=9, "pH值"=10, "溶解氧"=11, "电导率"=12, "浊度"=13, "叶绿素a"=14, "藻密度"=15, "蓝绿藻"=16, "氧化还原电位"=17, "溶解氧%"=18, "盐度"=19] ("站号")
            n271 = call "多参数控制命令.vi"("控制命令"=w531, "站号"=w532) -> ("error out"=w534:errorcluster)  [unwired: 9 in]
            n272 = case shown="无错误" w534 {
              tunnel: ["启动成功" ("消息") "启动失败" ("消息")] -> w533
              frame No Error {
              }
              frame Error {
              }
            }
            n273 = One Button Dialog(message=w533) -> ()  [unwired: 1 in, 1 out]
          }
        }
      }
      event "停止测量(全部)": Value Change {
        n274 = event-data() -> ()  [unwired: 1 in, 6 out]
        n275 = property class="Bool (严格)"(reference=w538) -> ("Value"=w537:bool)  [unwired: 1 in, 2 out]
        n276 = case shown="真" w537 {
          frame False {
            n277 = One Button Dialog(message="启动失败，请先通电" ("消息")) -> ()  [unwired: 1 in, 1 out]
          }
          frame True {
            w542 = u16 11 items=["启动测量（全部）"=1, "初始化（清洗）"=10, "停止测量（全部）"=11, "校时"=13, "启动测量（单个传感器）"=19, "停止测量（单个传感器）"=20] ("控制命令")
            w543 = u16 9 items=["氨氮"=3, "水温"=9, "pH值"=10, "溶解氧"=11, "电导率"=12, "浊度"=13, "叶绿素a"=14, "藻密度"=15, "蓝绿藻"=16, "氧化还原电位"=17, "溶解氧%"=18, "盐度"=19] ("站号")
            n278 = call "多参数控制命令.vi"("控制命令"=w542, "站号"=w543) -> ("error out"=w541:errorcluster)  [unwired: 9 in]
            n279 = case shown="错误" w541 {
              tunnel: ["停止成功" ("消息") "停止失败" ("消息")] -> w540
              frame No Error {
              }
              frame Error {
              }
            }
            n280 = One Button Dialog(message=w540) -> ()  [unwired: 1 in, 1 out]
          }
        }
      }
      event "初始化(清洗)": Value Change {
        n281 = event-data() -> ()  [unwired: 1 in, 6 out]
        n282 = property class="Bool (严格)"(reference=w547) -> ("Value"=w546:bool)  [unwired: 1 in, 2 out]
        n283 = case shown="真" w546 {
          frame False {
            n284 = One Button Dialog(message="启动失败，请先通电" ("消息")) -> ()  [unwired: 1 in, 1 out]
          }
          frame True {
            w551 = u16 10 items=["启动测量（全部）"=1, "初始化（清洗）"=10, "停止测量（全部）"=11, "校时"=13, "启动测量（单个传感器）"=19, "停止测量（单个传感器）"=20] ("控制命令")
            w552 = u16 9 items=["氨氮"=3, "水温"=9, "pH值"=10, "溶解氧"=11, "电导率"=12, "浊度"=13, "叶绿素a"=14, "藻密度"=15, "蓝绿藻"=16, "氧化还原电位"=17, "溶解氧%"=18, "盐度"=19] ("站号")
            n285 = call "多参数控制命令.vi"("控制命令"=w551, "站号"=w552) -> ("error out"=w549:errorcluster)  [unwired: 9 in]
            n286 = case shown="错误" w549 {
              tunnel: ["初始化成功" ("消息") "初始化失败" ("消息")] -> w550
              frame No Error {
              }
              frame Error {
              }
            }
            n287 = One Button Dialog(message=w550) -> ()  [unwired: 1 in, 1 out]
          }
        }
      }
      event "启动测量(单探)": Value Change {
        n288 = event-data() -> ()  [unwired: 1 in, 6 out]
        n289 = property class="Bool (严格)"(reference=w556) -> ("Value"=w555:bool)  [unwired: 1 in, 2 out]
        n290 = property class="Ring (严格)"(reference=w558) -> ("Value"=w557:u16)  [unwired: 1 in, 2 out]
        n291 = case shown="真" w555 {
          tunnel: w557 -> [_ w560]
          frame False {
            n292 = One Button Dialog(message="启动失败，请先通电" ("消息")) -> ()  [unwired: 1 in, 1 out]
          }
          frame True {
            w561 = u16 19 items=["启动测量（全部）"=1, "初始化（清洗）"=10, "停止测量（全部）"=11, "校时"=13, "启动测量（单个传感器）"=19, "停止测量（单个传感器）"=20] ("控制命令")
            n293 = call "多参数控制命令.vi"("控制命令"=w561, "站号"=w560) -> ("error out"=w563:errorcluster)  [unwired: 9 in]
            n294 = case shown="无错误" w563 {
              tunnel: ["启动成功" ("消息") "启动失败" ("消息")] -> w562
              frame No Error {
              }
              frame Error {
              }
            }
            n295 = One Button Dialog(message=w562) -> ()  [unwired: 1 in, 1 out]
          }
        }
      }
      event "停止测量(单探)": Value Change {
        n296 = event-data() -> ()  [unwired: 1 in, 6 out]
        n297 = property class="Bool (严格)"(reference=w567) -> ("Value"=w566:bool)  [unwired: 1 in, 2 out]
        n298 = property class="Ring (严格)"(reference=w569) -> ("Value"=w568:u16)  [unwired: 1 in, 2 out]
        n299 = case shown="真" w566 {
          tunnel: w568 -> [_ w571]
          frame False {
            n300 = One Button Dialog(message="启动失败，请先通电" ("消息")) -> ()  [unwired: 1 in, 1 out]
          }
          frame True {
            w572 = u16 20 items=["启动测量（全部）"=1, "初始化（清洗）"=10, "停止测量（全部）"=11, "校时"=13, "启动测量（单个传感器）"=19, "停止测量（单个传感器）"=20] ("控制命令")
            n301 = call "多参数控制命令.vi"("控制命令"=w572, "站号"=w571) -> ("error out"=w574:errorcluster)  [unwired: 9 in]
            n302 = case shown="错误" w574 {
              tunnel: ["停止成功" ("消息") "停止失败" ("消息")] -> w573
              frame No Error {
              }
              frame Error {
              }
            }
            n303 = One Button Dialog(message=w573) -> ()  [unwired: 1 in, 1 out]
          }
        }
      }
      event "写入KB": Value Change {
        n304 = event-data() -> ()  [unwired: 1 in, 6 out]
        n305 = property class="DigNum (严格)"(reference=w580) -> ("Value"=w579:dbl)  [unwired: 1 in, 2 out]
        n306 = property class="DigNum (严格)"(reference=w582) -> ("Value"=w581:dbl)  [unwired: 1 in, 2 out]
        n307 = property class="Bool (严格)"(reference=w578) -> ("Value"=w577:bool)  [unwired: 1 in, 2 out]
        n308 = property class="Ring (严格)"(reference=w584) -> ("Value"=w583:u16)  [unwired: 1 in, 2 out]
        n309 = case shown="假" w577 {
          tunnel: w583 -> [_ w590]
          tunnel: w581 -> [_ w589]
          tunnel: w579 -> [_ w588]
          frame False {
            n310 = One Button Dialog(message="启动失败，请先通电" ("消息")) -> ()  [unwired: 1 in, 1 out]
          }
          frame True {
            n311 = call "多参数校准写入.vi"("B"=w589, "K"=w588, "站号"=w590) -> ("error out"=w586:errorcluster)  [unwired: 8 in]
            n312 = case shown="错误" w586 {
              tunnel: ["写入成功" ("消息") "写入失败" ("消息")] -> w587
              frame No Error {
              }
              frame Error {
              }
            }
            n313 = One Button Dialog(message=w587) -> ()  [unwired: 1 in, 1 out]
          }
        }
      }
      event "K", "B": Mouse Down {
        n314 = event-data() -> ("CtlRef"=w596:refnum<vi>)  [unwired: 1 in, 5 out]
        n315 = property class="DigNum (严格)"(reference=w596) -> (reference out=w595:refnum<vi>, "Value"=w594:dbl)  [unwired: 1 in, 1 out]
        n316 = call "数字键盘.vi"("OldNumber"=w594) -> ("NewNumber"=w593:sgl)
        n317 = property class="DigNum (严格)"(reference=w595, "Value"=w593) -> ()  [unwired: 1 in, 2 out]
      }
      event "读取KB": Value Change {
        n318 = event-data() -> ()  [unwired: 1 in, 6 out]
        n319 = property class="Bool (严格)"(reference=w598) -> ("Value"=w597:bool)  [unwired: 1 in, 2 out]
        n320 = property class="Ring (严格)"(reference=w600) -> ("Value"=w599:u16)  [unwired: 1 in, 2 out]
        n321 = case shown="真" w597 {
          tunnel: w599 -> [_ w604]
          frame False {
            n322 = One Button Dialog(message="启动失败，请先通电" ("消息")) -> ()  [unwired: 1 in, 1 out]
          }
          frame True {
            n323 = call "多参校准读取.vi"("站号"=w604) -> ("error out"=w602:errorcluster, "B"=→"B":dbl, "K"=→"K":dbl)  [unwired: 8 in]
            n324 = case shown="无错误" w602 {
              tunnel: ["读取成功" ("消息") "读取失败" ("消息")] -> w603
              frame No Error {
              }
              frame Error {
              }
            }
            n325 = One Button Dialog(message=w603) -> ()  [unwired: 1 in, 1 out]
          }
        }
      }
      event "自动校准": Value Change {
        n326 = event-data() -> ()  [unwired: 1 in, 6 out]
        n327 = property class="Bool (严格)"(reference=w610) -> ("Value"=w609:bool)  [unwired: 1 in, 2 out]
        n328 = case shown="真" w609 {
          frame False {
            n329 = One Button Dialog(message="启动失败，请先通电" ("消息")) -> ()  [unwired: 1 in, 1 out]
          }
          frame True {
            n330 = call "多参校准.vi"() -> ()  [unwired: 12 in]
          }
        }
      }
      event "手动通电": Value Change {
        n331 = event-data() -> ("NewVal"=w613:bool)  [unwired: 1 in, 5 out]
        n332 = Boolean To (0,1)(Boolean=w613) -> (0, 1=w612:i16)
        n333 = Bundle By Name(cluster=T11 {"starting address"=0, "holding register value"=0}, "starting address"=u16 302, "holding register value"=w612) -> (w615:T11)
        n334 = call "采配水通讯指令.vi"("数据"=w615, "命令"=T12."单个写入") -> ()  [unwired: 10 in]
      }
    }
  }
